vi "运维调试_五参数.vi"(11 "编号":string) -> ()   [LabVIEW 2016, in "斯坦道多参数.lvlib"]
uses:
  <vilib>/Utility/miscctls.llb/LVPointTypeDef.ctl
  <vilib>/Plasmionique/MB Master/MB_Master/MB_Master.lvclass
  <vilib>/Utility/config.llb/NI_LVConfig.lvlib
panel:
  in  "仪器参数":bool
  in  "参数设置选项卡":enum32{"选项卡 1", "选项卡 2"}(tab)
  in  "pH":bool
  in  "DO":bool
  in  "Turb":bool
  in  "Cond":bool
  in  "Temp":bool
  in  "叶绿素a启用":bool
  in  "藻密度":bool
  in  "pH探头选择":u16(ring) items=["YL型", "MQ型", "NAQ型"]
  in  "DO探头选择":u16(ring) items=["YL型", "MQ型", "NAQ型"]
  in  "电导率探头选择":u16(ring) items=["YL型", "MQ型", "NAQ型"]
  in  "浊度探头选择":u16(ring) items=["YL型", "MQ型", "NAQ型"]
  in  "叶绿素a探头选择":u16(ring) items=["YL型", "MQ型", "NAQ型"]
  in  "藻密度探头选择":u16(ring) items=["YL型", "MQ型", "NAQ型"]
  in  "ORP启用":bool
  in  "ORP探头选择":u16(ring) items=["YL型", "MQ型", "NAQ型"]
  in  "校准选择":T1
  out "模块版本号":string
  out "权限等级":string
  in  "水样测量时间":dbl caption="水样测量时间:"
  in  "打开modbus":bool
  out "选项卡控件":enum32{"选项卡 1", "选项卡 2"}(tab)
  in  "VISA资源名称":refnum<visa-resource-name> caption="串口"
  in  "IP":string="localhost" caption="IP:"
  in  "Port":u16=502 caption="Port:"
  in  "自动断线重连":bool=TRUE
  in  "连接方式":u16(ring) items=["Modbus RTU", "Modbus TCP"]
  in  "密码锁":bool
  in  "设置页返回":bool
  in  "周期设置":bool
  out "当前串口":string
  out "运行状态":enum16{"空闲", "水样测试", "标样核查"}(ring)
  in  "停止":bool
  in  "标样核查":bool
  in  "水样测试":bool
  in  "设置":bool
  in  "探头校正返回":bool
  in  "探头校正":bool
  out "检测值":T2
  # "请设置仪器连接方式"
  # "请选择要启用的参数"
  # "min"
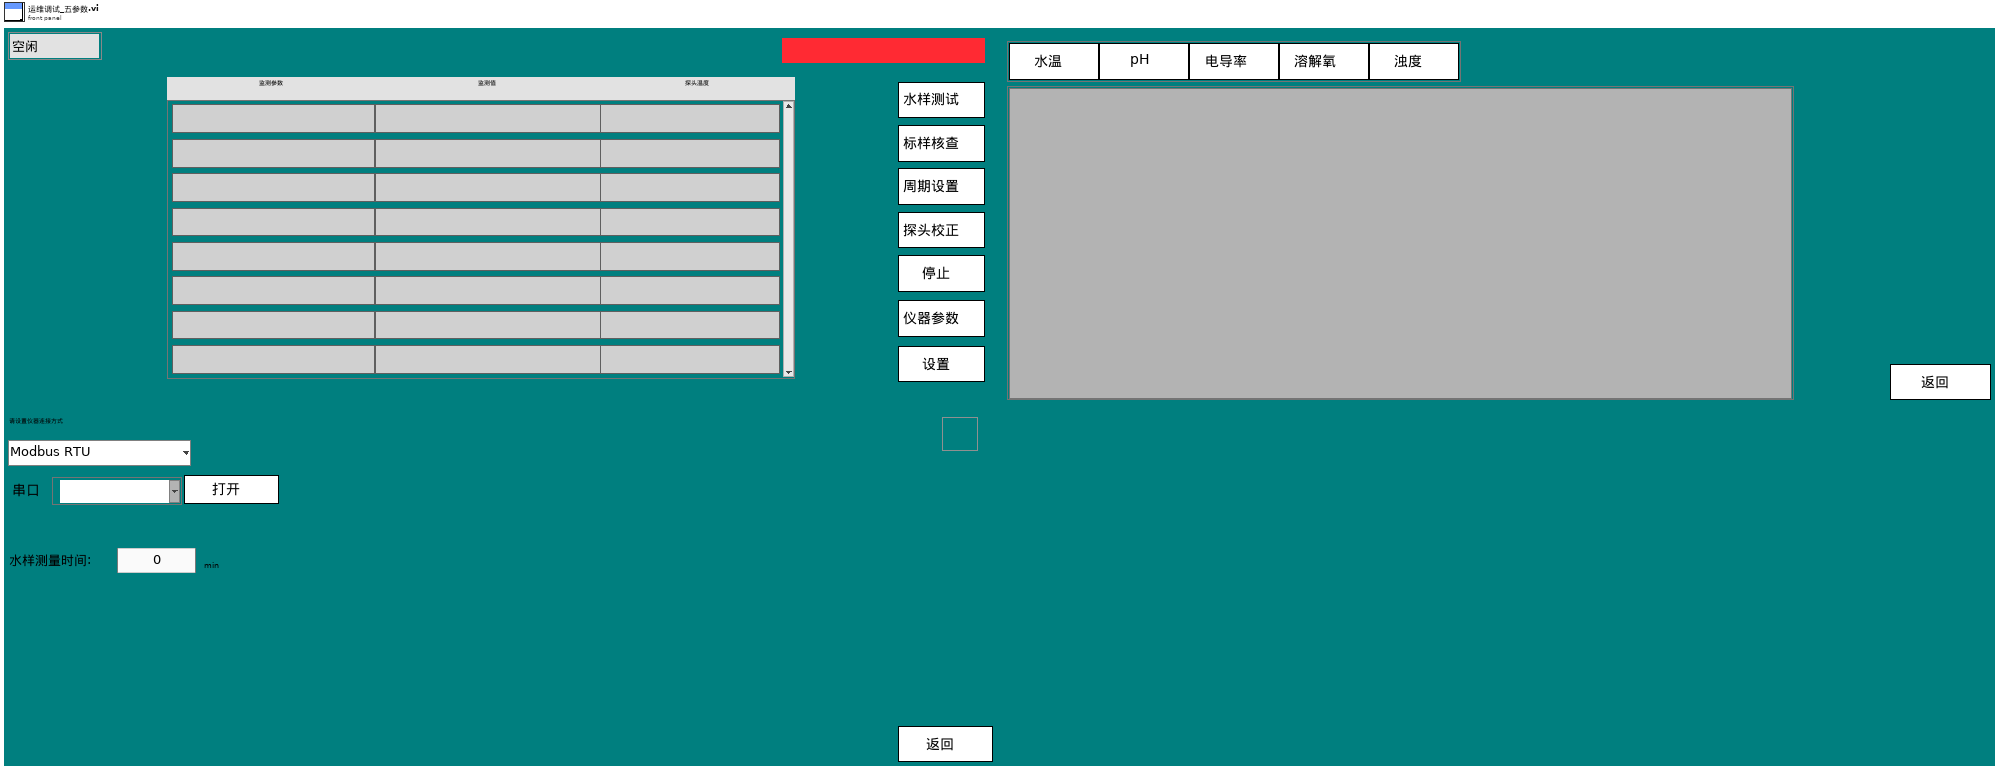
[diagram p1: front panel]
types:
  T1 = cluster{"水温校准":bool, "pH校准":bool, "电导率校准":bool, "溶解氧校准":bool, "浊度校准":bool, "叶绿素a校准":bool, "藻密度校准":bool, "ORP校准":bool}
  T2 = typedef "斯坦道多参数.lvlib/检测值.ctl" = cluster{"监测参数1":string, "浓度1":string, "探头温度1":string}[]
  T3 = typedef "LVPointTypeDef.ctl" = cluster{"Horizontal":i16, "Vertical":i16}
  T4 = cluster{"CH":u16, "监测值":dbl, "温度偏移修正值":sgl, "信号值":sgl}
  T5 = cluster{"温度测量值":sgl, "测量值":sgl, "温度偏移修正值":sgl, "信号值":sgl}
  T6 = cluster{"温度测量值":sgl, "DO%":sgl, "DOmg/L":sgl, "温度偏移修正值":sgl}
  T7 = cluster{"电极状态标志":u16, "电极型号标志":u16, "浊度测量值":sgl, "温度测量值":sgl, "浊度信号值":sgl, "浊度偏移修正值":sgl, "温度偏移修正值":sgl, "手动温度补偿值":sgl, "浊度电极零点":sgl, "浊度电极斜率":sgl, "第1点标准值记录":sgl, "第1点信号值记录":sgl, "第1点温度值记录":sgl, "第2点标准值记录":sgl, "第2点信号值记录":sgl, "第2点温度值记录":sgl, "命令滤波设定":u16, "温度模式":enum16{"ATC", "MTC"}, "生产批次":u16, "电极序号":u16, "串口地址":u16, "串口波特率":enum16{"9600", "19200", "115200"}, "串口校验位":enum16{"NONE", "ODD", "EVEN"}, "串口停止位":enum16{"1bit", "2bit"}, "第一点标准值":sgl, "第二点标准值":sgl, "第三点标准值":sgl}
  T8 = cluster{"电极状态标志":u16, "电极型号标志":u16, "溶解氧测量值":sgl, "温度测量值":sgl, "溶解氧饱和度值":sgl, "盐度补偿值":sgl, "大气压补偿值":sgl, "溶解氧偏移修正值":sgl, "温度偏移修正值":sgl, "手动温度补偿值":sgl, "溶解氧电极零点":sgl, "溶解氧电极斜率":sgl, "第1点标准值记录":sgl, "第1点信号值记录":sgl, "第1点温度值记录":sgl, "第2点标准值记录":sgl, "第2点信号值记录":sgl, "第2点温度值记录":sgl, "命令滤波设定":u16, "温度模式":enum16{"ATC", "MTC"}, "生产批次":u16, "电极序号":u16, "串口地址":u16, "串口波特率":enum16{"9600", "19200", "115200"}, "串口校验位":enum16{"NONE", "ODD", "EVEN"}, "串口停止位":enum16{"1bit", "2bit"}, "第一点标准值":sgl, "第二点标准值":sgl}
  T9 = cluster{"电极状态标志":u16, "电极型号标志":u16, "酸碱度测量值":sgl, "温度测量值":sgl, "酸碱度信号值":sgl, "温度信号值":sgl, "酸碱度偏移修正值":sgl, "温度偏移修正值":sgl, "手动温度补偿值":sgl, "酸碱度电极零点":sgl, "酸碱度电极斜率":sgl, "第1点标准值记录":sgl, "第1点信号值记录":sgl, "第1点温度值记录":sgl, "第2点标准值记录":sgl, "第2点信号值记录":sgl, "第2点温度值记录":sgl, "命令滤波设定":u16, "温度模式":enum16{"ATC", "MTC"}, "生产批次":u16, "电极序号":u16, "串口地址":u16, "串口波特率":enum16{"9600", "19200", "115200"}, "串口校验位":enum16{"NONE", "ODD", "EVEN"}, "串口停止位":enum16{"1bit", "2bit"}, "第一点标准值":sgl, "第二点标准值":sgl}
  T10 = cluster{"测量量程":dbl, "测量精度":dbl, "测量间隔":dbl, "消解温度":dbl, "消解时长":dbl, "空白校准时间":timestamp, "曲线截距":dbl, "曲线斜率":dbl, "测量检出限":dbl, "测量信号值":dbl, "线性相关系数":dbl, "二次多项式系数":dbl, "标样校准时间":timestamp, "稀释倍数":dbl, "三项式系数":dbl, "空白标定系数":dbl, "量程系数":dbl, "F0/ORPA":dbl, "F1/ORPB":dbl, "F2/ORPK":dbl, "F3":dbl, "F4":dbl, "F5":dbl, "F6":dbl, "F7":dbl, "X0/滴定数":dbl, "量程":dbl}
  T11 = cluster{"电极状态标志":u16, "电极型号标志":u16, "电导率测量值":sgl, "温度测量值":sgl, "电导率信号值":sgl, "温度信号值":sgl, "温度补偿系数":sgl, "电导率偏移修正值":sgl, "温度偏移修正值":sgl, "手动温度补偿值":sgl, "电导率电极零点":sgl, "电导率电极斜率":sgl, "命令滤波设定":u16, "温度模式":enum16{"ATC", "MTC"}, "生产批次":u16, "电极序号":u16, "串口地址":u16, "串口波特率":enum16{"9600", "19200", "115200"}, "串口校验位":enum16{"NONE", "ODD", "EVEN"}, "串口停止位":enum16{"1bit", "2bit"}, "第一点标准值":sgl, "第二点标准值":sgl}
  T12 = enum8{"Enabled", "Disabled", "Disabled and Grayed Out"}
  T13 = cluster{"pH探头选择":u16, "DO探头选择":u16, "电导率探头选择":u16, "浊度探头选择":u16, "叶绿素a探头选择":u16, "蓝绿藻探头选择":u16, "orp探头选择":u16}
  T14 = cluster{"监测参数1":string, "浓度1":string, "探头温度1":string}[]
  T15 = cluster{"周期设置类型":enum16{"定点启动", "间隔启动"}, "定时功能启用":bool, "定时间隔":u32, "24H周期设置":bool[]}
  T16 = enum32{"Bad", "Idle", "Run top level", "Running"}
  T17 = typedef "LVDateTimeRec.ctl" = cluster{"秒数的小数部分":dbl, "秒":i32, "分":i32, "时":i32, "日":i32, "月":i32, "年":i32, "天数（周）":i32, "天数（年）":i32, "DST":i32}
  T18 = cluster{"Major":u16, "Minor":u16, "Fix":u16, "Build":u16}
  T19 = typedef "NI_LVConfig.lvlib/Config Data RefNum.ctl" = refnum<k1>
  T20 = cluster{"baud rate (bps)":u32, "stop bits":u16, "parity":u16, "flow control":u16, "timeout":u32, "retries":i32}
  T21 = cluster{"pH校准VI引用句柄":refnum<vi>, "DO校准VI引用句柄":refnum<vi>, "COND校准VI引用句柄":refnum<vi>, "TURB校准VI引用句柄":refnum<vi>, "CHLA校准VI引用句柄":refnum<vi>, "BGA校准VI引用句柄":refnum<vi>, "ORP校准VI引用句柄":refnum<vi>}
  T22 = cluster{"测量量程":dbl, "测量精度":dbl, "测量间隔":dbl, "消解温度":dbl, "消解时长":dbl, "空白校准时间":timestamp, "曲线截距":dbl, "曲线斜率":dbl, "测量检出限":dbl, "测量信号值":dbl, "线性相关系数":dbl, "二次多项式系数":dbl, "标样校准时间":timestamp, "稀释倍数":dbl, "三项式系数":dbl, "空白标定系数":dbl, "量程系数":dbl, "F0/ORPA":dbl, "F1/ORPB":dbl, "F2/ORPK":dbl, "F3":dbl, "F4":dbl, "F5":dbl, "F6":dbl, "F7":dbl, "X0/滴定数":dbl, "量程":dbl}[]
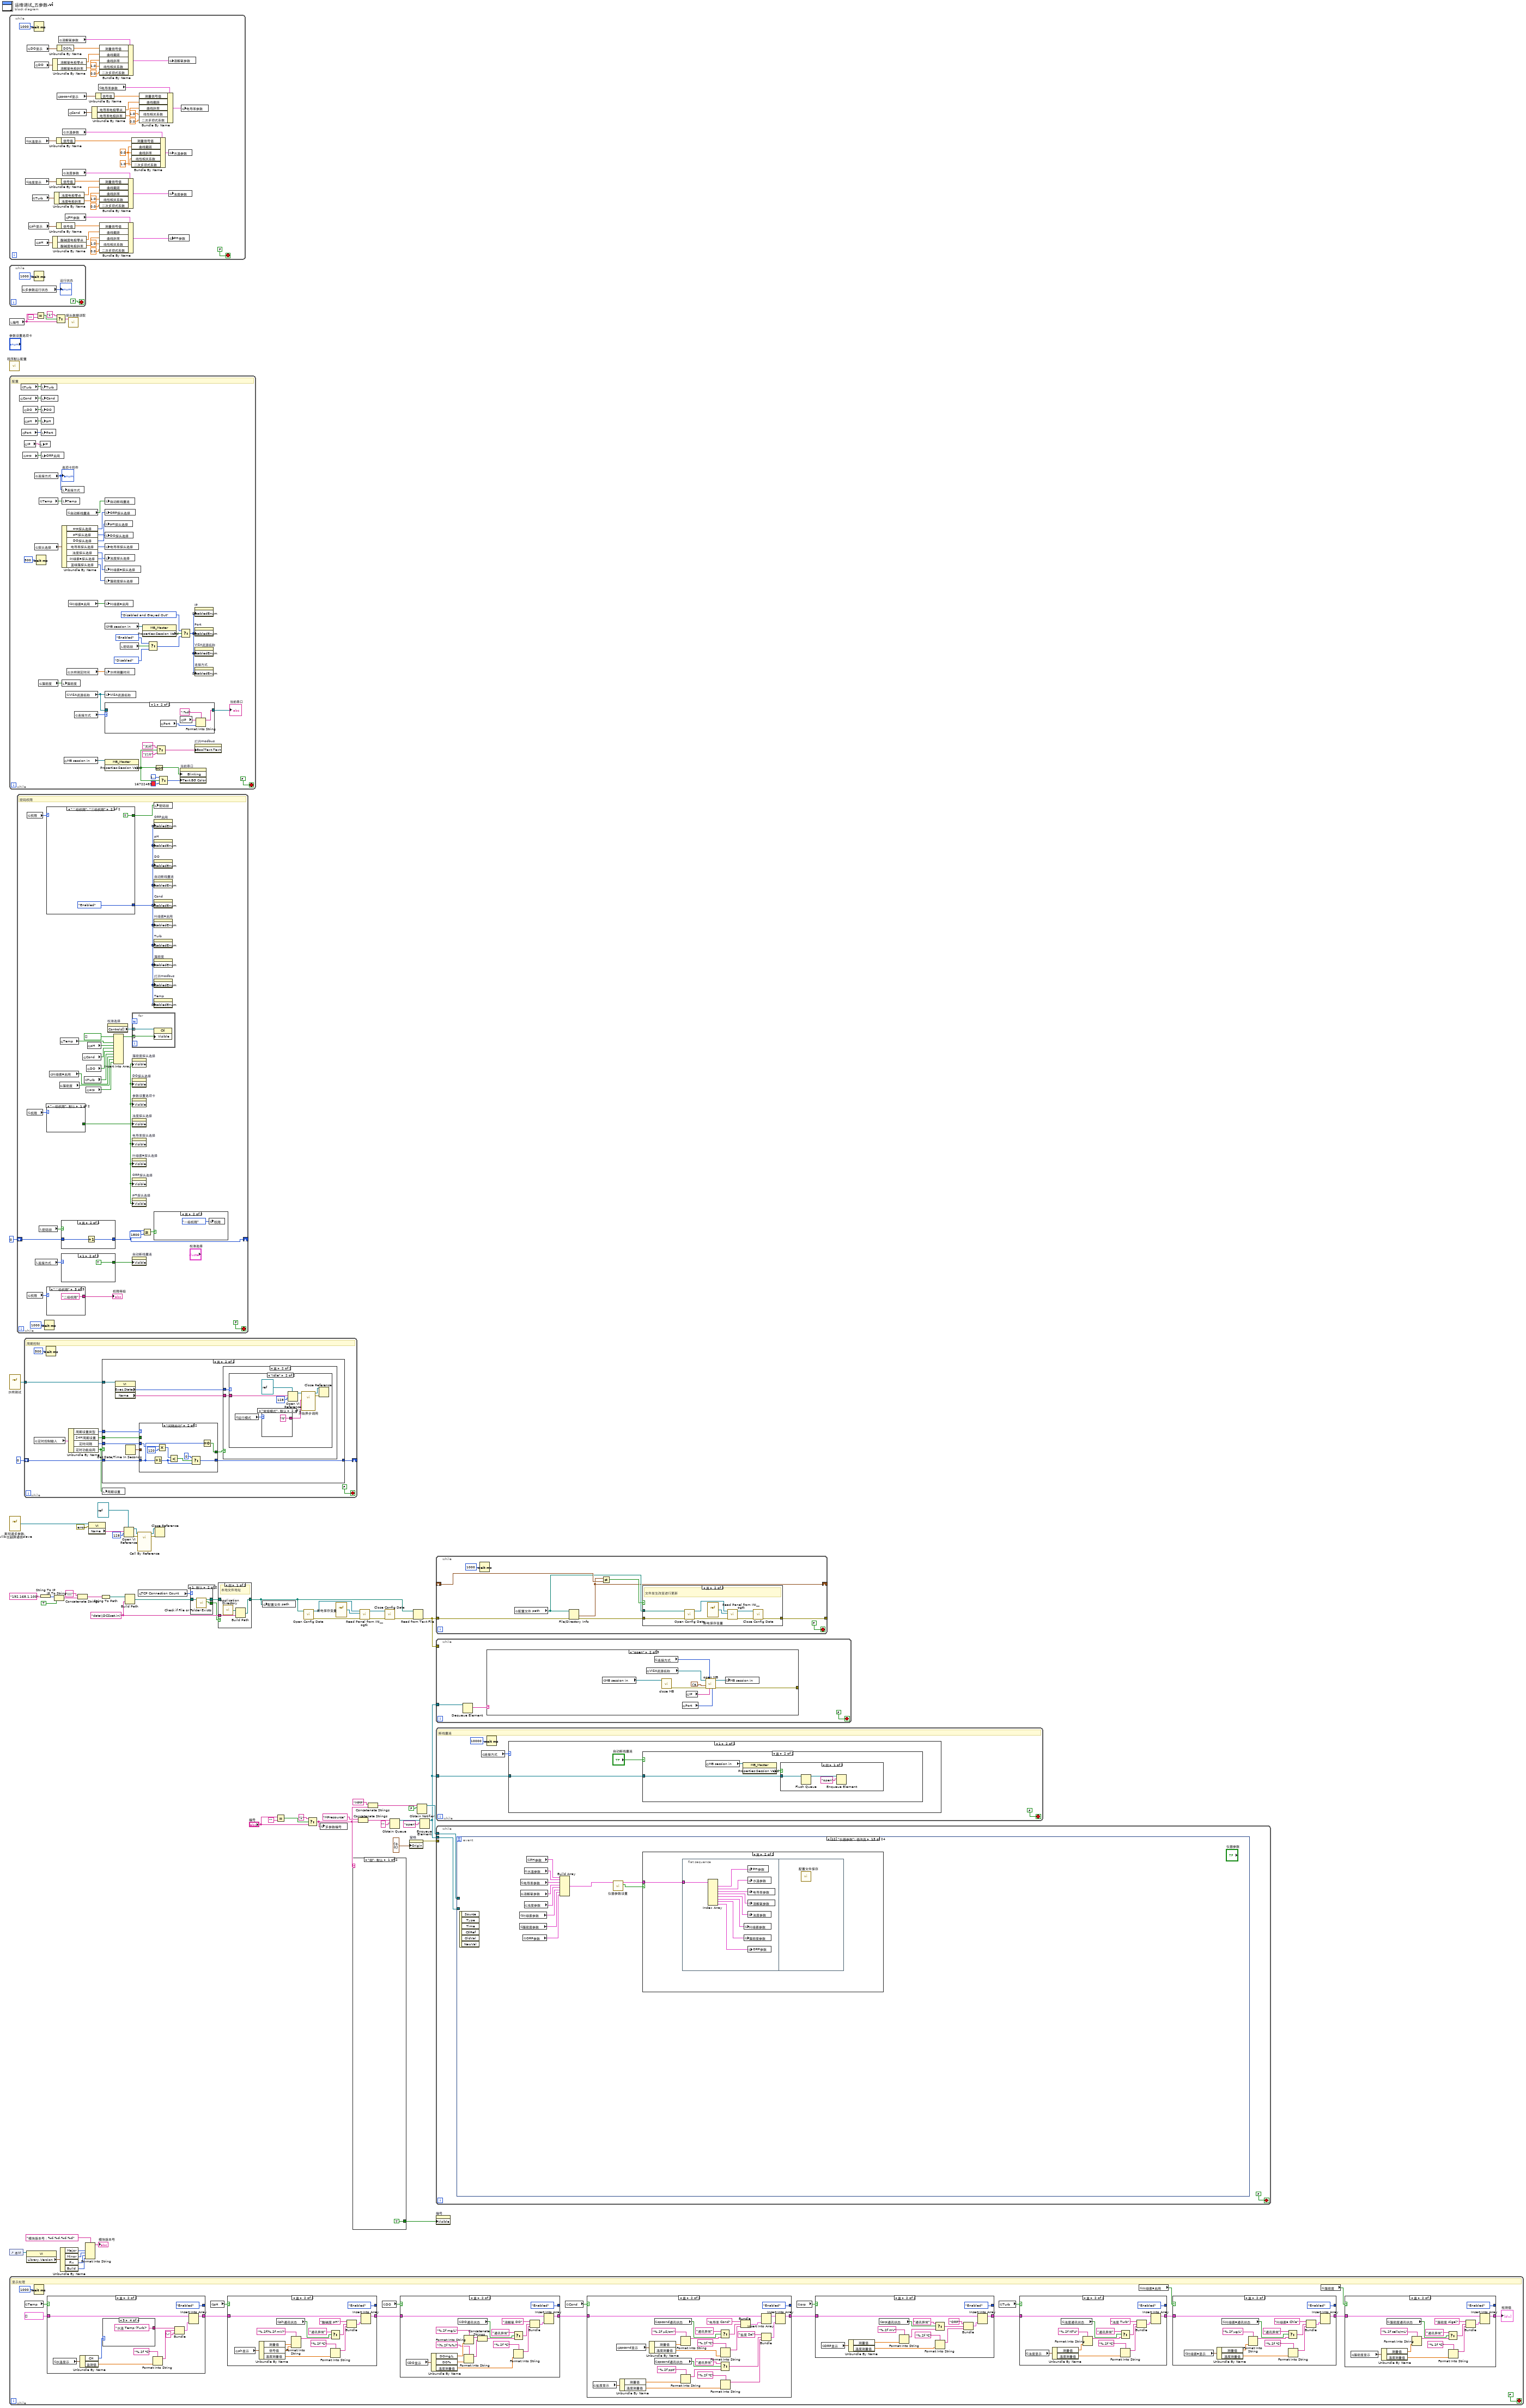
[diagram p0: block diagram]
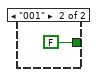
[diagram p3: hidden frame]
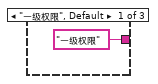
[diagram p12: hidden frame]
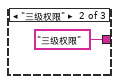
[diagram p13: hidden frame]
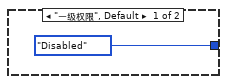
[diagram p14: hidden frame]
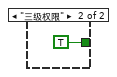
[diagram p15: hidden frame]
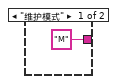
[diagram p19: hidden frame]
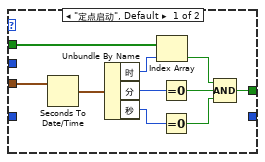
[diagram p20: hidden frame]
diagram:
  w34 = "data\\DCSset.ini" ("名称或相对路径")
  n1 = while {
    stop <- FALSE stop-if-true
    w64 = 0.0 ("二次多项式系数")
    n2 = global read "多参数全局变量.vi" "水温显示"() -> (w85:T4)
    n3 = global read "多参数全局变量.vi" "浊度显示"() -> (w67:T5)
    n4 = global read "多参数全局变量.vi" "DO显示"() -> (w99:T6)
    n5 = global read "多参数全局变量.vi" "ph显示"() -> (w94:T5)
    n6 = global read "国弘过程全局变量.vi" "Turb"() -> (w69:T7)
    n7 = Wait (ms)(milliseconds to wait=u32 1000 ("等待时间（毫秒）")) -> ()  [unwired: 1 out]
    n8 = global read "国弘过程全局变量.vi" "DO"() -> (w101:T8)
    n9 = global read "国弘过程全局变量.vi" "pH"() -> (w92:T9)
    n10 = Unbundle By Name(w101) -> ("溶解氧电极零点"=w102:sgl, "溶解氧电极斜率"=w103:sgl)
    n11 = Unbundle By Name(w92) -> ("酸碱度电极零点"=w91:sgl, "酸碱度电极斜率"=w90:sgl)
    n12 = Unbundle By Name(w69) -> ("浊度电极零点"=w70:sgl, "浊度电极斜率"=w71:sgl)
    n13 = Unbundle By Name(w85) -> ("信号值"=w86:sgl)
    n14 = Unbundle By Name(w67) -> ("信号值"=w68:sgl)
    n15 = Unbundle By Name(w94) -> ("信号值"=w93:sgl)
    n16 = Unbundle By Name(w99) -> ("DO%"=w100:sgl)
    n17 = global read "多参数全局变量.vi" "spcond显示"() -> (w80:T5)
    n18 = global read "断电保存变量.vi" "溶解氧参数"() -> (w97:T10)
    n19 = global read "断电保存变量.vi" "水温参数"() -> (w83:T10)
    n20 = global read "断电保存变量.vi" "浊度参数"() -> (w65:T10)
    n21 = global read "断电保存变量.vi" "PH参数"() -> (w96:T10)
    n22 = global read "国弘过程全局变量.vi" "Cond"() -> (w78:T11)
    n23 = Unbundle By Name(w78) -> ("电导率电极零点"=w77:sgl, "电导率电极斜率"=w76:sgl)
    n24 = Unbundle By Name(w80) -> ("信号值"=w79:sgl)
    n25 = global read "断电保存变量.vi" "电导率参数"() -> (w82:T10)
    n26 = Bundle By Name(cluster=w97, "测量信号值"=w100, "曲线截距"=w102, "曲线斜率"=w103, "线性相关系数"=1.0, "二次多项式系数"=0.0) -> (w98:T10)
    n27 = Bundle By Name(cluster=w65, "测量信号值"=w68, "曲线截距"=w70, "曲线斜率"=w71, "线性相关系数"=1.0, "二次多项式系数"=0.0) -> (w66:T10)
    n28 = Bundle By Name(cluster=w96, "测量信号值"=w93, "曲线截距"=w91, "曲线斜率"=w90, "线性相关系数"=1.0, "二次多项式系数"=0.0) -> (w95:T10)
    n29 = Bundle By Name(cluster=w83, "测量信号值"=w86, "曲线截距"=w64, "曲线斜率"=w64, "线性相关系数"=1.0, "二次多项式系数"=w64) -> (w84:T10)
    n30 = Bundle By Name(cluster=w82, "测量信号值"=w79, "曲线截距"=w77, "曲线斜率"=w76, "线性相关系数"=1.0, "二次多项式系数"=0.0) -> (w81:T10)
    n31 = global write "断电保存变量.vi" "溶解氧参数"(w98) -> ()
    n32 = global write "断电保存变量.vi" "水温参数"(w84) -> ()
    n33 = global write "断电保存变量.vi" "浊度参数"(w66) -> ()
    n34 = global write "断电保存变量.vi" "PH参数"(w95) -> ()
    n35 = global write "断电保存变量.vi" "电导率参数"(w81) -> ()
  }
  n36 = while {
    stop <- FALSE stop-if-true
    n37 = global read "多参数全局变量.vi" "多参数运行状态"() -> (→"运行状态":u16)
    n38 = Wait (ms)(milliseconds to wait=u32 1000 ("等待时间（毫秒）")) -> ()  [unwired: 1 out]
  }
  n39 = local read "编号"() -> (w10:string)
  n40 = call "程序默认配置.vi"() -> ()  [unwired: 11 in, 1 out]
  n41 = while {
    stop <- FALSE stop-if-true
    # "配置"
    n42 = global read "断电保存变量.vi" "Cond"() -> (w149:bool)
    n43 = global read "断电保存变量.vi" "Turb"() -> (w148:bool)
    n44 = global read "断电保存变量.vi" "Port"() -> (w127:u16)
    n45 = global read "断电保存变量.vi" "orp"() -> (w112:bool)
    n46 = global read "断电保存变量.vi" "DO"() -> (w150:bool)
    n47 = global read "断电保存变量.vi" "pH"() -> (w151:bool)
    n48 = global read "断电保存变量.vi" "IP"() -> (w128:string)
    n49 = global read "断电保存变量.vi" "连接方式"() -> (w120:u16)
    "选项卡控件" <- w120
    n50 = global read "断电保存变量.vi" "探头选择"() -> (w138:T13)
    n51 = Wait (ms)(milliseconds to wait=u32 500 ("等待时间（毫秒）")) -> ()  [unwired: 1 out]
    n52 = global read "断电保存变量.vi" "藻密度"() -> (w146:bool)
    n53 = global read "断电保存变量.vi" "Temp"() -> (w152:bool)
    n54 = local write "IP"(w128) -> ()
    n55 = local write "Turb"(w148) -> ()
    n56 = local write "Cond"(w149) -> ()
    n57 = local write "DO"(w150) -> ()
    n58 = local write "pH"(w151) -> ()
    n59 = local write "Port"(w127) -> ()
    n60 = local write "ORP启用"(w112) -> ()
    n61 = local write "连接方式"(w120) -> ()
    n62 = local write "Temp"(w152) -> ()
    n63 = Unbundle By Name(w138) -> ("orp探头选择"=w111:u16, "pH探头选择"=w121:u16, "DO探头选择"=w137:u16, "电导率探头选择"=w136:u16, "浊度探头选择"=w135:u16, "叶绿素a探头选择"=w134:u16, "蓝绿藻探头选择"=w133:u16)
    n64 = local write "藻密度"(w146) -> ()
    n65 = global read "多参数全局变量.vi" "MB session in"() -> (w142:refnum<class "MB_Master.lvclass">)
    n66 = global read "断电保存变量.vi" "VISA资源名称"() -> (w124:refnum<visa-resource-name>)
    n67 = global read "断电保存变量.vi" "自动断线重连"() -> (w115:bool)
    n68 = global read "断电保存变量.vi" "水样测定时间"() -> (w114:dbl)
    n69 = global read "断电保存变量.vi" "叶绿素a启用"() -> (w147:bool)
    n70 = global read "断电保存变量.vi" "连接方式"() -> (w125:u16)
    n71 = local write "自动断线重连"(w115) -> ()
    n72 = local write "ORP探头选择"(w111) -> ()
    n73 = local write "pH探头选择"(w121) -> ()
    n74 = local write "DO探头选择"(w137) -> ()
    n75 = local write "电导率探头选择"(w136) -> ()
    n76 = local write "浊度探头选择"(w135) -> ()
    n77 = local write "叶绿素a探头选择"(w134) -> ()
    n78 = local write "藻密度探头选择"(w133) -> ()
    n79 = local write "叶绿素a启用"(w147) -> ()
    n80 = global read "多参数全局变量.vi" "MB session in"() -> (w145:refnum<class "MB_Master.lvclass">)
    n81 = local write "水样测量时间"(w114) -> ()
    n82 = local write "VISA资源名称"(w124) -> ()
    n83 = case shown="1" w125 {
      tunnel: w124 -> [w154 _]
      tunnel: [w154 w155] -> w123
      frame 0, Default {
      }
      frame 1 {
        n84 = global read "断电保存变量.vi" "Port"() -> (w156:u16)
        n85 = global read "断电保存变量.vi" "IP"() -> (w158:string)
        n86 = Format Into String(format string=":%d" ("格式字符串"), initial string=w158, w156) -> (resulting string=w155:string)  [unwired: 1 in, 1 out]
      }
    }
    "当前串口" <- w123
    n87 = property class="MB_Master"(reference=w142) -> ("Properties:Session Valid"=w119:bool)  [unwired: 1 in, 2 out]
    n88 = local read "密码锁"() -> (w132:bool)
    n89 = property class="MB_Master"(reference=w145) -> ("Properties:Session Valid"=w144:bool)  [unwired: 1 in, 2 out]
    n90 = Select(t=T12."Enabled" ("f"), s=w132, f=T12."Disabled") -> (s? t:f=w130:T12)
    n91 = Not(x=w119) -> (.not. x?=w122:bool)
    n92 = Select(t="关闭" ("布尔文本.文本"), s=w119, f="打开" ("布尔文本.文本")) -> (s? t:f=w139:string)
    n93 = Select(t=u32 16777216, s=w119, f=u32 16722483) -> (s? t:f=w116:u32)
    n94 = property on="当前串口" class="Str"("Blinking"=w122, "Text.BG Color"=w116) -> ()  [unwired: 2 in, 2 out]
    n95 = Select(t=T12."Disabled and Grayed Out" ("禁用"), s=w144, f=w130) -> (s? t:f=w126:T12)
    n96 = property on="IP" class="Str"("DisabledEnum"=w126) -> ()  [unwired: 2 in, 2 out]
    n97 = property on="Port" class="DigNum (严格)"("DisabledEnum"=w126) -> ()  [unwired: 2 in, 2 out]
    n98 = property on="VISA资源名称" class="VISAName"("DisabledEnum"=w126) -> ()  [unwired: 2 in, 2 out]
    n99 = property on="连接方式" class="Ring (严格)"("DisabledEnum"=w126) -> ()  [unwired: 2 in, 2 out]
    n100 = property on="打开modbus" class="Bool"("BoolText.Text"=w139) -> ()  [unwired: 2 in, 2 out]
  }
  n101 = vi-ref "水样测试.vi"() -> (w53:refnum<vi>)
  n102 = vi-ref "斯坦道多参数.lvlib:主副屏通信slave.vi"() -> (w35:refnum<vi>)
  n103 = control-ref of="本VI"() -> (w26:refnum<vi>)
  n104 = while {
    stop <- FALSE stop-if-true
    # "显示处理"
    n105 = global read "断电保存变量.vi" "Temp"() -> (w175:bool)
    n106 = Wait (ms)(milliseconds to wait=u32 1000 ("等待时间（毫秒）")) -> ()  [unwired: 1 out]
    n107 = case shown="真" w175 {
      tunnel: [w316 w321] -> w172
      tunnel: T14 [] ("数组") -> [w316 w322]
      tunnel: [T12."Disabled and Grayed Out" ("禁用") T12."Enabled" ("禁用")] -> _
      frame False {
      }
      frame True {
        n108 = global read "多参数全局变量.vi" "水温显示"() -> (w319:T4)
        n109 = Unbundle By Name(w319) -> ("CH"=w318:u16, "监测值"=w317:dbl)
        n110 = case shown="3" w318 {
          tunnel: ["水温 Temp (pH)" ("监测参数1") "水温 Temp (Cond)" ("监测参数1") "水温 Temp (DO)" ("监测参数1") "水温 Temp (Turb)" ("监测参数1")] -> w326
          frame 0, Default {
          }
          frame 1 {
          }
          frame 2 {
          }
          frame 3 {
          }
        }
        n111 = Format Into String(format string="%.2f ℃" ("格式字符串"), w317) -> (resulting string=w325:string)  [unwired: 2 in, 1 out]
        n112 = Bundle("监测参数1"=w326, w325, "探头温度1"="-") -> (w323:cluster{"监测参数1":string, string, "探头温度1":string})  [unwired: 1 in]
        n113 = Insert Into Array(array=w322, new element=w323) -> (w321:T14)  [unwired: 1 in]
      }
    }
    n114 = global read "断电保存变量.vi" "pH"() -> (w173:bool)
    n115 = case shown="真" w173 {
      tunnel: [w298 w306] -> w170
      tunnel: w172 -> [w298 w308]
      tunnel: [T12."Disabled and Grayed Out" ("禁用") T12."Enabled" ("禁用")] -> _
      frame False {
      }
      frame True {
        n116 = global read "多参数全局变量.vi" "ph显示"() -> (w304:T5)
        n117 = Unbundle By Name(w304) -> ("测量值"=w314:sgl, "信号值"=w299:sgl, "温度测量值"=w312:sgl)
        n118 = global read "多参数全局变量.vi" "ph通讯状态"() -> (w302:bool)
        n119 = Format Into String(format string="%.2f(%.2f mV)" ("格式字符串"), w314, w299) -> (resulting string=w301:string)  [unwired: 2 in, 1 out]
        n120 = Select(t="通讯异常" ("格式字符串"), s=w302, f=w301) -> (s? t:f=w300:string)
        n121 = Format Into String(format string="%.2f ℃" ("格式字符串"), w312) -> (resulting string=w310:string)  [unwired: 2 in, 1 out]
        n122 = Bundle("监测参数2"="酸碱度 pH", "格式字符串"=w300, w310) -> (w307:cluster{"监测参数2":string, "格式字符串":string, string})  [unwired: 1 in]
        n123 = Insert Into Array(array=w308, new element=w307) -> (w306:T14)  [unwired: 1 in]
      }
    }
    n124 = global read "断电保存变量.vi" "DO"() -> (w171:bool)
    n125 = case shown="真" w171 {
      tunnel: [w277 w284] -> w167
      tunnel: w170 -> [w277 w285]
      tunnel: [T12."Disabled and Grayed Out" ("禁用") T12."Enabled" ("禁用")] -> _
      frame False {
      }
      frame True {
        n126 = global read "多参数全局变量.vi" "DO显示"() -> (w282:T6)
        n127 = Unbundle By Name(w282) -> ("DOmg/L"=w293:sgl, "DO%"=w291:sgl, "温度测量值"=w295:sgl)
        n128 = global read "多参数全局变量.vi" "DO通讯状态"() -> (w280:bool)
        n129 = Format Into String(format string="%.2f mg/L" ("格式字符串"), w293) -> (resulting string=w290:string)  [unwired: 2 in, 1 out]
        n130 = Format Into String(format string="(%.2f %%)" ("格式字符串"), w291) -> (resulting string=w289:string)  [unwired: 2 in, 1 out]
        n131 = Concatenate Strings(w290, w289) -> (w279:string)
        n132 = Select(t="通讯异常" ("格式字符串"), s=w280, f=w279) -> (s? t:f=w278:string)
        n133 = Format Into String(format string="%.2f ℃" ("格式字符串"), w295) -> (resulting string=w287:string)  [unwired: 2 in, 1 out]
        n134 = Bundle("监测参数2"="溶解氧 DO", "格式字符串"=w278, w287) -> (w286:cluster{"监测参数2":string, "格式字符串":string, string})  [unwired: 1 in]
        n135 = Insert Into Array(array=w285, new element=w286) -> (w284:T14)  [unwired: 1 in]
      }
    }
    n136 = global read "断电保存变量.vi" "Cond"() -> (w169:bool)
    n137 = case shown="真" w169 {
      tunnel: w167 -> [w247 w271]
      tunnel: [w247 w260] -> w159
      tunnel: [T12."Disabled and Grayed Out" ("禁用") T12."Enabled" ("禁用")] -> _
      frame False {
      }
      frame True {
        n138 = global read "多参数全局变量.vi" "盐度显示"() -> (w253:T5)
        n139 = global read "多参数全局变量.vi" "spcond显示"() -> (w268:T5)
        n140 = Unbundle By Name(w253) -> ("测量值"=w254:sgl, "温度测量值"=w255:sgl)
        n141 = Unbundle By Name(w268) -> ("测量值"=w267:sgl, "温度测量值"=w266:sgl)
        n142 = global read "多参数全局变量.vi" "spcond通讯状态"() -> (w264:bool)
        n143 = global read "多参数全局变量.vi" "spcond通讯状态"() -> (w257:bool)
        n144 = Format Into String(format string="%.2f μS/cm" ("格式字符串"), w267) -> (resulting string=w263:string)  [unwired: 2 in, 1 out]
        n145 = Format Into String(format string="%.2f ppt" ("格式字符串"), w254) -> (resulting string=w258:string)  [unwired: 2 in, 1 out]
        n146 = Select(t="通讯异常" ("格式字符串"), s=w264, f=w263) -> (s? t:f=w262:string)
        n147 = Select(t="通讯异常" ("格式字符串"), s=w257, f=w258) -> (s? t:f=w259:string)
        n148 = Format Into String(format string="%.2f ℃" ("格式字符串"), w266) -> (resulting string=w272:string)  [unwired: 2 in, 1 out]
        n149 = Format Into String(format string="%.2f ℃" ("格式字符串"), w255) -> (resulting string=w252:string)  [unwired: 2 in, 1 out]
        n150 = Bundle("监测参数2"="电导率 Cond", "格式字符串"=w262, w272) -> (w270:cluster{"监测参数2":string, "格式字符串":string, string})  [unwired: 1 in]
        n151 = Insert Into Array(array=w271, new element=w270) -> (w261:T14)  [unwired: 1 in]
        n152 = Bundle("监测参数2"="盐度 Sal", "格式字符串"=w259, w252) -> (w248:cluster{"监测参数2":string, "格式字符串":string, string})  [unwired: 1 in]
        n153 = Insert Into Array(array=w261, new element=w248) -> (w260:T14)  [unwired: 1 in]
      }
    }
    n154 = global read "断电保存变量.vi" "orp"() -> (w161:bool)
    n155 = case shown="真" w161 {
      tunnel: w159 -> [w179 w190]
      tunnel: [w179 w188] -> w160
      tunnel: [T12."Disabled and Grayed Out" ("禁用") T12."Enabled" ("禁用")] -> _
      frame False {
      }
      frame True {
        n156 = global read "多参数全局变量.vi" "ORP显示"() -> (w186:T5)
        n157 = Unbundle By Name(w186) -> ("测量值"=w185:sgl, "温度测量值"=w184:sgl)
        n158 = global read "多参数全局变量.vi" "orp通讯状态"() -> (w182:bool)
        n159 = Format Into String(format string="%.2f mV" ("格式字符串"), w185) -> (resulting string=w181:string)  [unwired: 2 in, 1 out]
        n160 = Select(t="通讯异常" ("格式字符串"), s=w182, f=w181) -> (s? t:f=w180:string)
        n161 = Format Into String(format string="%.2f ℃" ("格式字符串"), w184) -> (resulting string=w191:string)  [unwired: 2 in, 1 out]
        n162 = Bundle("监测参数2"="ORP", "格式字符串"=w180, w191) -> (w189:cluster{"监测参数2":string, "格式字符串":string, string})  [unwired: 1 in]
        n163 = Insert Into Array(array=w190, new element=w189) -> (w188:T14)  [unwired: 1 in]
      }
    }
    n164 = global read "断电保存变量.vi" "Turb"() -> (w168:bool)
    n165 = case shown="真" w168 {
      tunnel: w160 -> [w230 w241]
      tunnel: [w230 w239] -> w166
      tunnel: [T12."Disabled and Grayed Out" ("禁用") T12."Enabled" ("禁用")] -> _
      frame False {
      }
      frame True {
        n166 = global read "多参数全局变量.vi" "浊度显示"() -> (w237:T5)
        n167 = Unbundle By Name(w237) -> ("测量值"=w236:sgl, "温度测量值"=w235:sgl)
        n168 = global read "多参数全局变量.vi" "浊度通讯状态"() -> (w233:bool)
        n169 = Format Into String(format string="%.2f NTU" ("格式字符串"), w236) -> (resulting string=w232:string)  [unwired: 2 in, 1 out]
        n170 = Select(t="通讯异常" ("格式字符串"), s=w233, f=w232) -> (s? t:f=w231:string)
        n171 = Format Into String(format string="%.2f ℃" ("格式字符串"), w235) -> (resulting string=w243:string)  [unwired: 2 in, 1 out]
        n172 = Bundle("监测参数2"="浊度 Turb", "格式字符串"=w231, w243) -> (w240:cluster{"监测参数2":string, "格式字符串":string, string})  [unwired: 1 in]
        n173 = Insert Into Array(array=w241, new element=w240) -> (w239:T14)  [unwired: 1 in]
      }
    }
    n174 = global read "断电保存变量.vi" "叶绿素a启用"() -> (w165:bool)
    n175 = case shown="真" w165 {
      tunnel: w166 -> [w213 w224]
      tunnel: [w213 w222] -> w163
      tunnel: [T12."Disabled and Grayed Out" ("禁用") T12."Enabled" ("禁用")] -> _
      frame False {
      }
      frame True {
        n176 = global read "多参数全局变量.vi" "叶绿素a显示"() -> (w218:T5)
        n177 = Unbundle By Name(w218) -> ("测量值"=w221:sgl, "温度测量值"=w220:sgl)
        n178 = global read "多参数全局变量.vi" "叶绿素a通讯状态"() -> (w216:bool)
        n179 = Format Into String(format string="%.2f μg/L" ("格式字符串"), w221) -> (resulting string=w215:string)  [unwired: 2 in, 1 out]
        n180 = Select(t="通讯异常" ("格式字符串"), s=w216, f=w215) -> (s? t:f=w214:string)
        n181 = Format Into String(format string="%.2f ℃" ("格式字符串"), w220) -> (resulting string=w226:string)  [unwired: 2 in, 1 out]
        n182 = Bundle("监测参数2"="叶绿素a Chla", "格式字符串"=w214, w226) -> (w223:cluster{"监测参数2":string, "格式字符串":string, string})  [unwired: 1 in]
        n183 = Insert Into Array(array=w224, new element=w223) -> (w222:T14)  [unwired: 1 in]
      }
    }
    n184 = global read "断电保存变量.vi" "藻密度"() -> (w164:bool)
    n185 = case shown="真" w164 {
      tunnel: w163 -> [w196 w207]
      tunnel: [w196 w205] -> w162
      tunnel: [T12."Disabled and Grayed Out" ("禁用") T12."Enabled" ("禁用")] -> _
      frame False {
      }
      frame True {
        n186 = global read "多参数全局变量.vi" "藻密度显示"() -> (w201:T5)
        n187 = Unbundle By Name(w201) -> ("测量值"=w204:sgl, "温度测量值"=w203:sgl)
        n188 = global read "多参数全局变量.vi" "藻密度通讯状态"() -> (w199:bool)
        n189 = Format Into String(format string="%.2f cells/mL" ("格式字符串"), w204) -> (resulting string=w198:string)  [unwired: 2 in, 1 out]
        n190 = Select(t="通讯异常" ("格式字符串"), s=w199, f=w198) -> (s? t:f=w197:string)
        n191 = Format Into String(format string="%.2f ℃" ("格式字符串"), w203) -> (resulting string=w209:string)  [unwired: 2 in, 1 out]
        n192 = Bundle("监测参数2"="藻密度 Algal", "格式字符串"=w197, w209) -> (w206:cluster{"监测参数2":string, "格式字符串":string, string})  [unwired: 1 in]
        n193 = Insert Into Array(array=w207, new element=w206) -> (w205:T14)  [unwired: 1 in]
      }
    }
    "检测值" <- w162
  }
  n194 = while {
    shift-right: [w354] -> _
    shift-left: u32 0 ("等待时间（毫秒）") -> [w355]
    stop <- FALSE stop-if-true
    # "密码权限"
    n195 = global read "多参数全局变量.vi" "权限"() -> (w345:enum16{"一级权限", "二级权限", "三级权限"})
    n196 = global read "多参数全局变量.vi" "权限"() -> (w346:enum16{"一级权限", "二级权限", "三级权限"})
    n197 = global read "多参数全局变量.vi" "权限"() -> (w347:enum16{"一级权限", "二级权限", "三级权限"})
    n198 = local read "连接方式"() -> (w351:u16)
    n199 = local read "密码锁"() -> (w356:bool)
    n200 = Wait (ms)(milliseconds to wait=u32 1000 ("等待时间（毫秒）")) -> ()  [unwired: 1 out]
    n201 = case shown="\"二级权限\", \"三级权限\"" w345 {
      tunnel: [T12."Disabled" ("禁用") T12."Enabled" ("禁用")] -> w349
      tunnel: [_ TRUE ("可见")] -> w344
      frame "一级权限", Default {
      }
      frame "二级权限", "三级权限" {
      }
    }
    n202 = case shown="\"一级权限\", 默认" w346 {
      tunnel: [_ TRUE ("可见")] -> w332
      frame "一级权限", Default {
      }
      frame "三级权限" {
      }
    }
    n203 = case shown="\"二级权限\"" w347 {
      tunnel: ["一级权限" ("权限等级") "三级权限" ("权限等级") "二级权限" ("权限等级")] -> w348
      frame "一级权限", Default {
      }
      frame "三级权限" {
      }
      frame "二级权限" {
      }
    }
    "权限等级" <- w348
    n204 = global read "断电保存变量.vi" "叶绿素a启用"() -> (w336:bool)
    n205 = global read "断电保存变量.vi" "藻密度"() -> (w335:bool)
    n206 = global read "断电保存变量.vi" "Temp"() -> (w342:bool)
    n207 = case shown="真" w356 {
      tunnel: w355 -> [_ w364]
      tunnel: [_ w363] -> w354
      frame False {
      }
      frame True {
        n208 = Increment(x=w364) -> (x+1=w363:u32)
      }
    }
    n209 = case shown="1" w351 {
      tunnel: [_ TRUE ("可见")] -> w350
      frame 0, Default {
      }
      frame 1 {
      }
    }
    n210 = global read "断电保存变量.vi" "Cond"() -> (w339:bool)
    n211 = global read "断电保存变量.vi" "Turb"() -> (w337:bool)
    n212 = global read "断电保存变量.vi" "orp"() -> (w334:bool)
    n213 = global read "断电保存变量.vi" "DO"() -> (w338:bool)
    n214 = global read "断电保存变量.vi" "pH"() -> (w340:bool)
    n215 = property on="校准选择" class="Clust"() -> ("Controls[]"=w343:refnum<vi>[])  [unwired: 2 in, 2 out]
    n216 = Insert Into Array(array=bool[] [] ("数组"), new element #1=w342, new element #2=w340, new element #3=w339, new element #4=w338, new element #5=w337, new element #6=w336, new element #7=w335, new element #8=w334) -> (w333:bool[])  [unwired: 1 in]
    n217 = for {
      tunnel: w343 -> [w360] mode=indexing
      tunnel: w333 -> [w359] mode=indexing
      n218 = property class="Ctl"(reference=w360, "Visible"=w359) -> ()  [unwired: 1 in, 2 out]
    }
    n219 = property on="藻密度探头选择" class="Ring (严格)"("Visible"=w332) -> ()  [unwired: 2 in, 2 out]
    n220 = property on="DO探头选择" class="Ring (严格)"("Visible"=w332) -> ()  [unwired: 2 in, 2 out]
    n221 = property on="参数设置选项卡" class="TabCtl (严格)"("Visible"=w332) -> ()  [unwired: 2 in, 2 out]
    n222 = property on="浊度探头选择" class="Ring (严格)"("Visible"=w332) -> ()  [unwired: 2 in, 2 out]
    n223 = property on="电导率探头选择" class="Ring (严格)"("Visible"=w332) -> ()  [unwired: 2 in, 2 out]
    n224 = property on="叶绿素a探头选择" class="Ring (严格)"("Visible"=w332) -> ()  [unwired: 2 in, 2 out]
    n225 = property on="ORP探头选择" class="Ring (严格)"("Visible"=w332) -> ()  [unwired: 2 in, 2 out]
    n226 = property on="pH探头选择" class="Ring (严格)"("Visible"=w332) -> ()  [unwired: 2 in, 2 out]
    n227 = property on="自动断线重连" class="Bool (严格)"("Visible"=w350) -> ()  [unwired: 2 in, 2 out]
    n228 = Greater Or Equal?(x=w354, y=u32 1800) -> (x >= y?=w352:bool)
    n229 = local write "密码锁"(w344) -> ()
    n230 = property on="ORP启用" class="Bool (严格)"("DisabledEnum"=w349) -> ()  [unwired: 2 in, 2 out]
    n231 = property on="pH" class="Bool (严格)"("DisabledEnum"=w349) -> ()  [unwired: 2 in, 2 out]
    n232 = property on="DO" class="Bool (严格)"("DisabledEnum"=w349) -> ()  [unwired: 2 in, 2 out]
    n233 = property on="自动断线重连" class="Bool (严格)"("DisabledEnum"=w349) -> ()  [unwired: 2 in, 2 out]
    n234 = property on="Cond" class="Bool (严格)"("DisabledEnum"=w349) -> ()  [unwired: 2 in, 2 out]
    n235 = property on="叶绿素a启用" class="Bool (严格)"("DisabledEnum"=w349) -> ()  [unwired: 2 in, 2 out]
    n236 = property on="Turb" class="Bool (严格)"("DisabledEnum"=w349) -> ()  [unwired: 2 in, 2 out]
    n237 = property on="藻密度" class="Bool (严格)"("DisabledEnum"=w349) -> ()  [unwired: 2 in, 2 out]
    n238 = property on="打开modbus" class="Bool"("DisabledEnum"=w349) -> ()  [unwired: 2 in, 2 out]
    n239 = property on="Temp" class="Bool (严格)"("DisabledEnum"=w349) -> ()  [unwired: 2 in, 2 out]
    n240 = case shown="真" w352 {
      frame False {
      }
      frame True {
        n241 = global write "多参数全局变量.vi" "权限"(enum16{"一级权限", "二级权限", "三级权限"}."一级权限" ("权限")) -> ()
      }
    }
  }
  n242 = while {
    tunnel: w53 -> [w374]
    shift-right: [w373] -> _
    shift-left: u32 0 ("等待时间（毫秒）") -> [w375]
    stop <- FALSE stop-if-true
    # "周期控制"
    n243 = global read "断电保存变量.vi" "定时控制输入"() -> (w377:T15)
    n244 = Wait (ms)(milliseconds to wait=u32 500 ("等待时间（毫秒）")) -> ()  [unwired: 1 out]
    n245 = Unbundle By Name(w377) -> ("周期设置类型"=w379:enum16{"定点启动", "间隔启动"}, "24H周期设置"=w378:bool[], "定时间隔"=w376:u32, "定时功能启用"=w372:bool)
    n246 = case shown="真" w372 {
      tunnel: w379 -> [_ w390]
      tunnel: w378 -> [_ w389]
      tunnel: w376 -> [_ w387]
      tunnel: w375 -> [_ w383]
      tunnel: w374 -> [_ w386]
      tunnel: [_ w382] -> w373
      frame False {
      }
      frame True {
        n247 = property class="VI"(reference=w386) -> ("Exec.State"=w384:T16, "Name"=w385:string)  [unwired: 1 in, 2 out]
        n248 = Get Date/Time In Seconds() -> (seconds since 1Jan1904=w391:timestamp)
        n249 = case shown="\"间隔启动\"" w390 {
          tunnel: w391 -> [w413 _]
          tunnel: w389 -> [w410 _]
          tunnel: [w404 w421] -> w388
          tunnel: w387 -> [_ w420]
          tunnel: w383 -> [_ w422]
          tunnel: [_ w416] -> w382
          frame "定点启动", Default {
            n250 = Seconds To Date/Time(time stamp (now)=w413) -> (date time rec=w412:T17)  [unwired: 1 in]
            n251 = Unbundle By Name(w412) -> ("时"=w411:i32, "分"=w409:i32, "秒"=w408:i32)
            n252 = Index Array(array=w410, index=w411) -> (element=w407:bool)
            n253 = Equal To 0?(x=w409) -> (x = 0?=w406:bool)
            n254 = Equal To 0?(x=w408) -> (x = 0?=w405:bool)
            n255 = Compound Arithmetic op=AND ("复合运算")(w407, w406, w405) -> (w404:bool)
          }
          frame "间隔启动" {
            n256 = Increment(x=w422) -> (x+1=w415:u32)
            n257 = Multiply(x=w420, y=u32 120) -> (x*y=w414:u32)
            n258 = Less?(x=w414, y=w415) -> (x < y?=w418:bool)
            n259 = Select(t=u32 0 ("y"), s=w418, f=w415) -> (s? t:f=w416:u32)
            n260 = Equal To 0?(x=w422) -> (x = 0?=w421:bool)
          }
        }
        n261 = case shown="真" w388 {
          tunnel: w384 -> [_ w393]
          tunnel: w385 -> [_ w392]
          frame False {
          }
          frame True {
            n262 = case shown="\"Idle\"" w393 {
              tunnel: w392 -> [_ w398]
              frame "Bad", Default {
              }
              frame "Idle" {
                n263 = global read "多参数全局变量.vi" "运行模式"() -> (w396:enum16{"维护模式", "常规模式", "应急模式", "质控模式"})
                n264 = case shown="\"常规模式\", 默认" w396 {
                  tunnel: ["M" ("数据标记表") "N" ("数据标记表")] -> w395
                  frame "维护模式" {
                  }
                  frame "常规模式", Default {
                  }
                }
                n265 = Open VI Reference(type specifier VI Refnum (for type only)=refnum<vi> refnum, vi path=w398, options=128 ("选项")) -> (vi reference=w399:refnum<vi>)  [unwired: 3 in, 1 out]
                n266 = call-by-ref "开始异步调用"(reference=w399, "数据标记表"=w395) -> (reference out=w400:refnum<vi>, error out=w401:errorcluster)  [unwired: 12 in]
                n267 = Close Reference(reference=w400, error in (no error)=w401) -> ()  [unwired: 1 out]
              }
            }
          }
        }
      }
    }
    n268 = local write "周期设置"(w372) -> ()
  }
  n269 = property class="VI"(reference=w26) -> ("Library.Version"=w25:T18)  [unwired: 1 in, 2 out]
  n270 = Equal?(x=w10, y="") -> (x = y?=w12:bool)
  n271 = String To IP(1:"192.168.1.100" ("名称")) -> (0:w33:u32)
  n272 = IP To String(1:TRUE ("句点符号？(F)"), 2:w33) -> (0:w30:string)
  n273 = Select(t="1", s=w12, f=w10) -> (s? t:f=w9:string)
  n274 = Unbundle By Name(w25) -> ("Major"=w23:u16, "Minor"=w22:u16, "Fix"=w21:u16, "Build"=w20:u16)
  n275 = call "探头数据读取.vi"("编号"=w9) -> ()  [unwired: 11 in]
  n276 = Concatenate Strings("\\\\" ("字符串"), w30) -> (w31:string)
  n277 = Format Into String(format string="模块版本号：%d.%d.%d.%d" ("格式字符串"), w23, w22, w21, w20) -> (resulting string=→"模块版本号":string)  [unwired: 2 in, 1 out]
  n278 = property class="VI"(reference=w35, error in=errorcluster {"status"=FALSE, "code"=0, "source"=""} ("错误输出")) -> ("Name"=w36:string)  [unwired: 2 out]
  n279 = String To Path(string=w31) -> (path=w28:path)
  n280 = Open VI Reference(type specifier VI Refnum (for type only)=refnum<vi> refnum, vi path=w36, options=128 ("选项")) -> (vi reference=w38:refnum<vi>, error out=w40:errorcluster)  [unwired: 3 in]
  n281 = Build Path(base path=w28, name or relative path=w34) -> (appended path=w4:path)
  n282 = call-by-ref "?"(reference=w38, error in=w40) -> (reference out=w42:refnum<vi>, error out=w41:errorcluster)  [unwired: 12 in]
  n283 = global read "多参数全局变量.vi" "TCP Connection Count"() -> (w5:u32)
  n284 = Close Reference(reference=w42, error in (no error)=w41) -> ()  [unwired: 1 out]
  n285 = case shown="1, 默认" w5 {
    tunnel: w4 -> [w423 w426]
    tunnel: [w423 w425] -> w2
    tunnel: [_ w424] -> w3
    frame 0 {
    }
    frame 1, Default {
      n286 = call <vilib>:"Check if File or Folder Exists.vi"("path"=w426) -> ("file or folder exists?"=w424:bool, "dup path"=w425:path)  [unwired: 8 in, 1 out]
    }
  }
  n287 = case shown="假" w3 {
    tunnel: w2 -> [_ w430]
    tunnel: [w428 w430] -> w7
    tunnel: w34 -> [w427 _]
    frame False {
      # "本地文件地址"
      n288 = call <vilib>:"Application Directory.vi"() -> ("Application Directory"=w429:path)
      n289 = Build Path(base path=w429, name or relative path=w427) -> (appended path=w428:path)
    }
    frame True {
      # "网络共享地址"
    }
  }
  n290 = global write "多参数全局变量.vi" "配置文件 path"(w7) -> ()
  n291 = Equal?(x="编号", y="") -> (x = y?=w17:bool)
  n292 = call <vilib>:"Open Config Data.vi"("configuration file path"=w7) -> ("error out"=w47:errorcluster, "refnum"=w48:T19)  [unwired: 8 in, 1 out]
  n293 = Select(t="1", s=w17, f="编号") -> (s? t:f=w15:string)
  n294 = global write "多参数全局变量.vi" "多参数编号"(w15) -> ()
  n295 = vi-ref "断电保存变量.vi"() -> (w44:refnum<vi>)
  n296 = case shown="\"假\", 默认" w15 {
    tunnel: [TRUE ("可见") FALSE ("可见")] -> w27
    frame "假", Default {
    }
    frame "001" {
    }
  }
  n297 = Concatenate Strings("MPresource" ("名称（未命名）"), w15) -> (w55:string)
  n298 = call <userlib>:"Read Panel from INI__ogtk.vi"("error in (no error)"=w47, "VI ref"=w44, "refnum"=w48) -> ("error out"=w45:errorcluster, "refnum out"=w46:T19)  [unwired: 7 in]
  n299 = Concatenate Strings("MPP" ("名称（未命名）"), w15) -> (w56:string)
  n300 = call <vilib>:"Close Config Data.vi"("error in (no error)"=w45, "refnum"=w46) -> ("error out"=w8:errorcluster)  [unwired: 8 in, 1 out]
  n301 = Obtain Queue(name (unnamed)=w55, element data type="" ("名称（未命名）")) -> (queue out=w51:refnum<queue>)  [unwired: 3 in, 2 out]
  n302 = property on="窗格" class="Pane"("Origin"=T3 {"Horizontal"=0, "Vertical"=0} ("原点")) -> (error out=w63:errorcluster)  [unwired: 2 in, 1 out]
  n303 = Read from Text File(file (use dialog)=w7, error in=w8) -> (error out=w6:errorcluster)  [unwired: 2 in, 3 out]
  n304 = Obtain Notifier(name (unnamed)=w56, notification data type=FALSE) -> (notifier out=w59:refnum<notifier>)  [unwired: 2 in, 2 out]
  n305 = Enqueue Element(queue=w51, element="open" ("元素")) -> (queue out=w50:refnum<queue>)  [unwired: 2 in, 2 out]
  n306 = while {
    tunnel: [w440] -> _
    shift-right: [w433] -> _
    shift-left: _ -> [w438]
    tunnel: w6 -> [w435]
    stop <- FALSE stop-if-true
    n307 = Wait (ms)(milliseconds to wait=u32 1000 ("等待时间（毫秒）")) -> ()  [unwired: 1 out]
    n308 = global read "多参数全局变量.vi" "配置文件 path"() -> (w434:path)
    n309 = File/Directory Info(path=w434, error in=w435) -> (last mod=w433:timestamp, error out=w436:errorcluster)  [unwired: 5 out]
    n310 = Not Equal?(x=w433, y=w438) -> (x != y?=w437:bool)
    n311 = case shown="真" w437 {
      tunnel: [w442 w450] -> w440
      tunnel: w436 -> [w442 w449]
      tunnel: w434 -> [_ w443]
      frame False {
      }
      frame True {
        # "文件发生改变进行更新"
        n312 = call <vilib>:"Open Config Data.vi"("error in (no error)"=w449, "configuration file path"=w443) -> ("error out"=w448:errorcluster, "refnum"=w447:T19)  [unwired: 7 in, 1 out]
        n313 = vi-ref "断电保存变量.vi"() -> (w444:refnum<vi>)
        n314 = call <userlib>:"Read Panel from INI__ogtk.vi"("error in (no error)"=w448, "VI ref"=w444, "refnum"=w447) -> ("error out"=w446:errorcluster, "refnum out"=w445:T19)  [unwired: 7 in]
        n315 = call <vilib>:"Close Config Data.vi"("error in (no error)"=w446, "refnum"=w445) -> ("error out"=w450:errorcluster)  [unwired: 8 in, 1 out]
      }
    }
  }
  n316 = while {
    tunnel: w50 -> [w452]
    tunnel: w6 -> [_]
    stop <- FALSE stop-if-true
    n317 = Dequeue Element(queue=w452) -> (element=w451:string)  [unwired: 2 in, 3 out]
    n318 = case shown="\"open\"" w451 {
      tunnel: [_ w454 w464] -> _
      frame "假", Default {
      }
      frame "open" {
        n319 = global read "多参数全局变量.vi" "MB session in"() -> (w459:refnum<class "MB_Master.lvclass">)
        n320 = global read "断电保存变量.vi" "VISA资源名称"() -> (w461:refnum<visa-resource-name>)
        n321 = global read "断电保存变量.vi" "连接方式"() -> (w457:u16)
        n322 = call "close MB.vi"("MB session in"=w459) -> ("error out"=w462:errorcluster)  [unwired: 10 in]
        n323 = global read "断电保存变量.vi" "Port"() -> (w455:u16)
        n324 = global read "断电保存变量.vi" "IP"() -> (w456:string)
        n325 = call "open MB.vi"("Port (502)"=w455, "IP Address"=w456, "MODE"=w457, "error in (no error)"=w462, "Serial Config"=T20 {"baud rate (bps)"=9600, "stop bits"=10, "parity"=0, "flow control"=0, "timeout"=1000, "retries"=1}, "VISA资源名称"=w461) -> ("error out"=w454:errorcluster, "MB session out"=w458:refnum<class "MB_Master.lvclass">)  [unwired: 4 in]
        n326 = global write "多参数全局变量.vi" "MB session in"(w458) -> ()
      }
      frame "close" {
        n327 = global read "多参数全局变量.vi" "MB session in"() -> (w463:refnum<class "MB_Master.lvclass">)
        n328 = call "close MB.vi"("MB session in"=w463) -> ("error out"=w464:errorcluster)  [unwired: 10 in]
      }
    }
  }
  n329 = while {
    tunnel: w50 -> [w466]
    stop <- FALSE stop-if-true
    # "断线重连"
    n330 = global read "断电保存变量.vi" "连接方式"() -> (w467:u16)
    n331 = Wait (ms)(milliseconds to wait=u32 10000 ("等待时间（毫秒）")) -> ()  [unwired: 1 out]
    n332 = case shown="1" w467 {
      tunnel: w466 -> [_ w470]
      frame 0, Default {
      }
      frame 1 {
        n333 = case shown="真" "自动断线重连" {
          tunnel: w470 -> [_ w473]
          frame False {
          }
          frame True {
            n334 = global read "多参数全局变量.vi" "MB session in"() -> (w472:refnum<class "MB_Master.lvclass">)
            n335 = property class="MB_Master"(reference=w472) -> ("Properties:Session Valid"=w471:bool)  [unwired: 1 in, 2 out]
            n336 = case shown="假" w471 {
              tunnel: w473 -> [w474 _]
              frame False {
                n337 = Flush Queue(queue=w474) -> (queue out=w476:refnum<queue>)  [unwired: 1 in, 2 out]
                n338 = Enqueue Element(queue=w476, element="open" ("元素")) -> ()  [unwired: 2 in, 3 out]
              }
              frame True {
              }
            }
          }
        }
      }
    }
  }
  n339 = while {
    tunnel: w63 -> [_]
    tunnel: w59 -> [w478]
    tunnel: w50 -> [w477]
    stop <- FALSE stop-if-true
    n340 = event shown="[12] \"仪器参数\": 值改变" {
      selector: _ -> [_ _ _ _ _ _ _ _ _ _ _ _ _ _ _ _ _ _ _ _ _ _ _ _]
      dyn-events: _ -> [_ _ _ _ _ _ _ _ _ _ _ _ _ _ _ _ _ _ _ _ _ _ _ _]
      timeout: _ -> [_ _ _ _ _ _ _ _ _ _ _ _ _ _ _ _ _ _ _ _ _ _ _ _]
      tunnel: w478 -> [_ _ _ _ _ _ _ _ _ _ w580 _ _ _ _ _ _ _ _ _ _ _ _ _]
      tunnel: w477 -> [_ _ _ _ _ _ _ _ _ _ _ _ _ _ w618 _ _ _ _ _ _ _ _ _]
      event Timeout {
        n341 = event-data() -> ()  [unwired: 1 in, 3 out]
      }
      event "水样测量时间": Mouse Down {
        n342 = event-data() -> ("CtlRef"=w480:refnum<vi>)  [unwired: 1 in, 5 out]
        n343 = property class="DigNum (严格)"(reference=w480) -> (reference out=w483:refnum<vi>, "Value"=w482:dbl)  [unwired: 1 in, 1 out]
        n344 = call "数字键盘.vi"("OldNumber"=w482) -> ("NewNumber"=w481:dbl)  [unwired: 1 in]
        n345 = property class="DigNum (严格)"(reference=w483, "Val(Sgnl)"=w481) -> ()  [unwired: 1 in, 2 out]
      }
      event "pH探头选择", "DO探头选择", "电导率探头选择", "浊度探头选择", "叶绿素a探头选择", "藻密度探头选择", "ORP探头选择": Value Change {
        n346 = event-data() -> ("CtlRef"=w484:refnum<vi>, "NewVal"=w485:u16)  [unwired: 1 in, 4 out]
        n347 = Two Button Dialog(message="请再次确认修改的型号是否与实际匹配，否则将导致通讯异常，并且此操作将终止所有正在校准的参数！" ("消息")) -> (T button?=w486:bool)  [unwired: 2 in]
        n348 = case shown="真" w486 {
          tunnel: w485 -> [_ w489]
          tunnel: w484 -> [_ w488]
          frame False {
          }
          frame True {
            n349 = flat-sequence {
              tunnel: w489 -> [w490]
              tunnel: w488 -> [w494]
              frame #0 {
                n350 = property class="Ring (严格)"(reference=w494) -> ("Label.Text"=w493:string)  [unwired: 1 in, 2 out]
                n351 = global read "断电保存变量.vi" "探头选择"() -> (w492:T13)
                n352 = global read "多参数全局变量.vi" "校准VI引用句柄"() -> (w495:T21)
                n353 = case shown="\"ORP探头选择\"" w493 {
                  tunnel: w492 -> [w497 w500 w503 w506 w509 w512 w515 w518]
                  tunnel: [w497 w499 w502 w505 w508 w511 w514 w517] -> w491
                  tunnel: w490 -> [_ w498 w501 w504 w507 w510 w513 w516]
                  frame Default {
                  }
                  frame "pH探头选择" {
                    n354 = Bundle By Name(cluster=w500, "pH探头选择"=w498) -> (w499:T13)
                  }
                  frame "电导率探头选择" {
                    n355 = Bundle By Name(cluster=w503, "电导率探头选择"=w501) -> (w502:T13)
                  }
                  frame "DO探头选择" {
                    n356 = Bundle By Name(cluster=w506, "DO探头选择"=w504) -> (w505:T13)
                  }
                  frame "浊度探头选择" {
                    n357 = Bundle By Name(cluster=w509, "浊度探头选择"=w507) -> (w508:T13)
                  }
                  frame "叶绿素a探头选择" {
                    n358 = Bundle By Name(cluster=w512, "叶绿素a探头选择"=w510) -> (w511:T13)
                  }
                  frame "蓝绿藻探头选择" {
                    n359 = Bundle By Name(cluster=w515, "蓝绿藻探头选择"=w513) -> (w514:T13)
                  }
                  frame "ORP探头选择" {
                    n360 = Bundle By Name(cluster=w518, "蓝绿藻探头选择"=w516) -> (w517:T13)
                  }
                }
                n361 = Cluster To Array(cluster=w495) -> (array=w496:refnum<vi>[])
                n362 = for {
                  tunnel: w496 -> [w520] mode=indexing
                  tunnel: [w519] -> _ mode=indexing
                  n363 = invoke class="VI" method="Abort VI"(reference=w520) -> (error out=w519:errorcluster)  [unwired: 2 in, 2 out]
                }
                n364 = global write "断电保存变量.vi" "探头选择"(w491) -> ()
              }
              frame #1 {
                n365 = call "配置文件保存.vi"() -> ()  [unwired: 12 in]
              }
            }
          }
        }
      }
      event "VISA资源名称", "pH", "DO", "Turb", "Cond", "Temp", "叶绿素a启用", "打开modbus", "藻密度", "连接方式", "自动断线重连", "ORP启用": Mouse Down {
        n366 = event-data() -> ()  [unwired: 1 in, 6 out]
        n367 = local read "密码锁"() -> (w521:bool)
        n368 = case shown="假" w521 {
          frame False {
            n369 = One Button Dialog(message="当前操作权限不足,请提升权限!!!" ("消息")) -> ()  [unwired: 1 in, 1 out]
          }
          frame True {
          }
        }
      }
      event "IP": Mouse Down {
        n370 = event-data() -> ("CtlRef"=w524:refnum<vi>)  [unwired: 1 in, 7 out]
        n371 = property on="IP" class="Str"() -> ("DisabledEnum"=w523:T12)  [unwired: 2 in, 2 out]
        n372 = case shown="\"Disabled and Grayed Out\"" w523 {
          tunnel: w524 -> [w528 _ _]
          frame "Enabled" {
            n373 = property class="Str"(reference=w528) -> (reference out=w527:refnum<vi>, "Value"=w526:string)  [unwired: 1 in, 1 out]
            n374 = call "字符键盘.vi"("Old String"=w526) -> ("String"=w525:string)  [unwired: 10 in]
            n375 = property class="Str"(reference=w527, "Val(Sgnl)"=w525) -> ()  [unwired: 1 in, 2 out]
          }
          frame "Disabled and Grayed Out" {
            n376 = One Button Dialog(message="关闭连接后才可设置!" ("消息")) -> ()  [unwired: 1 in, 1 out]
          }
          frame "Disabled", Default {
            n377 = One Button Dialog(message="当前操作权限不足,请提升权限!!!" ("消息")) -> ()  [unwired: 1 in, 1 out]
          }
        }
      }
      event "Port": Mouse Down {
        n378 = event-data() -> ("CtlRef"=w532:refnum<vi>)  [unwired: 1 in, 7 out]
        n379 = property on="Port" class="DigNum (严格)"() -> ("DisabledEnum"=w531:T12)  [unwired: 2 in, 2 out]
        n380 = case shown="\"Enabled\"" w531 {
          tunnel: w532 -> [w536 _ _]
          frame "Enabled" {
            n381 = property class="DigNum (严格)"(reference=w536) -> (reference out=w535:refnum<vi>, "Value"=w534:u16)  [unwired: 1 in, 1 out]
            n382 = call "数字键盘.vi"("OldNumber"=w534) -> ("NewNumber"=w533:dbl)  [unwired: 1 in]
            n383 = property class="DigNum (严格)"(reference=w535, "Val(Sgnl)"=w533) -> ()  [unwired: 1 in, 2 out]
          }
          frame "Disabled and Grayed Out" {
            n384 = One Button Dialog(message="关闭连接后才可设置!" ("消息")) -> ()  [unwired: 1 in, 1 out]
          }
          frame "Disabled", Default {
            n385 = One Button Dialog(message="当前操作权限不足,请提升权限!!!" ("消息")) -> ()  [unwired: 1 in, 1 out]
          }
        }
      }
      event "密码锁": Value Change {
        n386 = event-data() -> ("NewVal"=w539:bool)  [unwired: 1 in, 5 out]
        n387 = case shown="假" w539 {
          frame False {
            n388 = global write "多参数全局变量.vi" "权限"(enum16{"一级权限", "二级权限", "三级权限"}."一级权限" ("权限")) -> ()
          }
          frame True {
            n389 = call "数字键盘.vi"("显示样式"=u32 2) -> ("NewNumber"=w544:dbl)  [unwired: 1 in]
            n390 = case shown="23506" w544 {
              tunnel: ["密码错误,即将切换为一级权限!" ("Infoin") "密码正确,即将切换为二级权限!" ("Infoin") "密码正确,即将切换为三级权限!" ("Infoin")] -> w543
              tunnel: [u32 16711680 ("颜色盒") _ _] -> w542
              tunnel: [enum16{"一级权限", "二级权限", "三级权限"}."一级权限" ("权限") enum16{"一级权限", "二级权限", "三级权限"}."二级权限" ("权限") enum16{"一级权限", "二级权限", "三级权限"}."三级权限" ("权限")] -> w541
              frame 0, Default {
              }
              frame 666 {
              }
              frame 23506 {
              }
            }
            n391 = global write "多参数全局变量.vi" "权限"(w541) -> ()
            n392 = call "TimeLmtDialog.vi"("颜色盒"=w542, "Infoin"=w543) -> ()  [unwired: 10 in]
          }
        }
      }
      event "周期设置": Mouse Down {
        n393 = event-data() -> ()  [unwired: 1 in, 6 out]
        n394 = flat-sequence {
          frame #0 {
            n395 = global read "断电保存变量.vi" "定时控制输入"() -> (w554:T15)
            n396 = call "周期设置.vi"("定时控制输入"=w554) -> ("定时控制输出"=w553:T15)  [unwired: 10 in]
            n397 = global write "断电保存变量.vi" "定时控制输入"(w553) -> ()
          }
          frame #1 {
            n398 = call "配置文件保存.vi"() -> ()  [unwired: 12 in]
          }
        }
      }
      event "水样测试": Value Change {
        n399 = event-data() -> ()  [unwired: 1 in, 6 out]
        n400 = vi-ref "水样测试.vi"() -> (w557:refnum<vi>)
        n401 = property class="VI"(reference=w557) -> ("Name"=w561:string, "Exec.State"=w559:T16)  [unwired: 1 in, 2 out]
        n402 = Open VI Reference(type specifier VI Refnum (for type only)=refnum<vi> refnum, vi path=w561, options=128 ("选项")) -> (vi reference=w562:refnum<vi>)  [unwired: 3 in, 1 out]
        n403 = case shown="\"Idle\"" w559 {
          tunnel: [w563 w566] -> w558
          tunnel: w562 -> [w563 w565]
          tunnel: "hd" ("数据标记表") -> [_ w564]
          frame "Bad", Default {
          }
          frame "Idle" {
            n404 = call-by-ref "开始异步调用"(reference=w565, "数据标记表"=w564) -> (reference out=w566:refnum<vi>)  [unwired: 12 in, 1 out]
          }
        }
        n405 = Close Reference(reference=w558) -> ()  [unwired: 1 in, 1 out]
      }
      event "标样核查": Value Change {
        n406 = event-data() -> ()  [unwired: 1 in, 6 out]
        n407 = call "标样核查配置.vi"() -> ("确认输出"=w567:bool)  [unwired: 11 in]
        n408 = case shown="真" w567 {
          frame False {
          }
          frame True {
            n409 = vi-ref "标样核查.vi"() -> (w569:refnum<vi>)
            n410 = property class="VI"(reference=w569) -> ("Name"=w573:string, "Exec.State"=w571:T16)  [unwired: 1 in, 2 out]
            n411 = Open VI Reference(type specifier VI Refnum (for type only)=refnum<vi> refnum, vi path=w573, options=128 ("选项")) -> (vi reference=w574:refnum<vi>)  [unwired: 3 in, 1 out]
            n412 = case shown="\"Idle\"" w571 {
              tunnel: [w575 w577] -> w570
              tunnel: w574 -> [w575 w576]
              frame "Bad", Default {
              }
              frame "Idle" {
                n413 = call-by-ref "开始异步调用"(reference=w576) -> (reference out=w577:refnum<vi>)  [unwired: 13 in, 1 out]
              }
            }
            n414 = Close Reference(reference=w570) -> ()  [unwired: 1 in, 1 out]
          }
        }
      }
      event "停止": Value Change {
        w578 = u16 3 items=["空闲", "水样测试", "标样核查", "停止"] ("主副屏同步启动")
        n415 = event-data() -> ()  [unwired: 1 in, 6 out]
        n416 = Send Notification(notification=TRUE ("通知"), notifier=w580) -> ()  [unwired: 1 in, 2 out]
        n417 = global write "多参数全局变量.vi" "主副屏同步启动"(w578) -> ()
      }
      event "设置": Value Change {
        n418 = event-data() -> ()  [unwired: 1 in, 6 out]
        n419 = property on="窗格" class="Pane"("Origin"=T3 {"Horizontal"=0, "Vertical"=628} ("原点")) -> ()  [unwired: 2 in, 2 out]
      }
      event "仪器参数": Value Change {
        n420 = event-data() -> ()  [unwired: 1 in, 6 out]
        n421 = global read "断电保存变量.vi" "叶绿素参数"() -> (w582:T10)
        n422 = global read "断电保存变量.vi" "藻密度参数"() -> (w583:T10)
        n423 = global read "断电保存变量.vi" "电导率参数"() -> (w590:T10)
        n424 = global read "断电保存变量.vi" "溶解氧参数"() -> (w588:T10)
        n425 = global read "断电保存变量.vi" "ORP参数"() -> (w584:T10)
        n426 = global read "断电保存变量.vi" "水温参数"() -> (w591:T10)
        n427 = global read "断电保存变量.vi" "浊度参数"() -> (w589:T10)
        n428 = global read "断电保存变量.vi" "PH参数"() -> (w592:T10)
        n429 = Build Array(w592, w591, w590, w588, w589, w582, w583, w584) -> (w587:T22)
        n430 = call "仪器参数设置.vi"("仪器参数设置输入"=w587) -> ("确定"=w586:bool, "仪器参数设置输出"=w585:T22)  [unwired: 9 in]
        n431 = case shown="真" w586 {
          tunnel: w585 -> [_ w593]
          frame False {
          }
          frame True {
            n432 = flat-sequence {
              tunnel: w593 -> [w602]
              frame #0 {
                n433 = Index Array(array=w602) -> (element #1=w600:T10, element #2=w599:T10, element #3=w597:T10, element #4=w598:T10, element #5=w601:T10, element #6=w596:T10, element #7=w594:T10, element #8=w595:T10)  [unwired: 8 in]
                n434 = global write "断电保存变量.vi" "叶绿素参数"(w596) -> ()
                n435 = global write "断电保存变量.vi" "藻密度参数"(w594) -> ()
                n436 = global write "断电保存变量.vi" "PH参数"(w600) -> ()
                n437 = global write "断电保存变量.vi" "水温参数"(w599) -> ()
                n438 = global write "断电保存变量.vi" "电导率参数"(w597) -> ()
                n439 = global write "断电保存变量.vi" "溶解氧参数"(w598) -> ()
                n440 = global write "断电保存变量.vi" "浊度参数"(w601) -> ()
                n441 = global write "断电保存变量.vi" "ORP参数"(w595) -> ()
              }
              frame #1 {
                n442 = call "配置文件保存.vi"() -> ()  [unwired: 12 in]
              }
            }
          }
        }
      }
      event "pH", "DO", "Turb", "Cond", "Temp", "叶绿素a启用", "藻密度", "VISA资源名称", "连接方式", "IP", "Port", "自动断线重连", "水样测量时间", "ORP启用": Value Change {
        n443 = event-data() -> ()  [unwired: 1 in, 6 out]
        n444 = flat-sequence {
          frame #0 {
            n445 = global write "断电保存变量.vi" "IP"("IP") -> ()
            n446 = global write "断电保存变量.vi" "藻密度"("藻密度") -> ()
            n447 = global write "断电保存变量.vi" "连接方式"("连接方式") -> ()
            n448 = global write "断电保存变量.vi" "Temp"("Temp") -> ()
            n449 = global write "断电保存变量.vi" "DO"("DO") -> ()
            n450 = global write "断电保存变量.vi" "Turb"("Turb") -> ()
            n451 = global write "断电保存变量.vi" "Port"("Port") -> ()
            n452 = global write "断电保存变量.vi" "pH"("pH") -> ()
            n453 = global write "断电保存变量.vi" "orp"("ORP启用") -> ()
            n454 = global write "断电保存变量.vi" "Cond"("Cond") -> ()
            n455 = global write "断电保存变量.vi" "叶绿素a启用"("叶绿素a启用") -> ()
            n456 = global write "断电保存变量.vi" "VISA资源名称"("VISA资源名称") -> ()
            n457 = global write "断电保存变量.vi" "水样测定时间"("水样测量时间") -> ()
            n458 = local read "自动断线重连"() -> (w605:bool)
            n459 = global write "断电保存变量.vi" "自动断线重连"(w605) -> ()
          }
          frame #1 {
            n460 = call "配置文件保存.vi"() -> ()  [unwired: 12 in]
          }
          frame #2 {
          }
        }
      }
      event "打开modbus": Value Change {
        n461 = event-data() -> ()  [unwired: 1 in, 6 out]
        n462 = global read "多参数全局变量.vi" "MB session in"() -> (w623:refnum<class "MB_Master.lvclass">)
        n463 = Flush Queue(queue=w618) -> (queue out=w617:refnum<queue>)  [unwired: 1 in, 2 out]
        n464 = property class="MB_Master"(reference=w623) -> ("Properties:Session Valid"=w622:bool)  [unwired: 1 in, 2 out]
        n465 = Select(t="close" ("元素"), s=w622, f="open" ("元素")) -> (s? t:f=w619:string)
        n466 = Enqueue Element(queue=w617, element=w619) -> ()  [unwired: 2 in, 3 out]
      }
      event "探头校正返回", "设置页返回": Value Change {
        n467 = event-data() -> ()  [unwired: 1 in, 6 out]
        n468 = property on="窗格" class="Pane"("Origin"=T3 {"Horizontal"=0, "Vertical"=0} ("原点")) -> ()  [unwired: 2 in, 2 out]
      }
      event "探头校正", "校准选择.水温校准": Value Change {
        n469 = event-data() -> ()  [unwired: 1 in, 6 out]
        n470 = property on="窗格" class="Pane"("Origin"=T3 {"Horizontal"=1656, "Vertical"=0} ("原点")) -> ()  [unwired: 2 in, 2 out]
        n471 = vi-ref "水温校准.vi"() -> (w625:refnum<vi>)
        n472 = property class="VI"(reference=w625) -> (reference out=w627:refnum<vi>, "Exec.State"=w626:T16)  [unwired: 1 in, 1 out]
        n473 = case shown="\"Bad\", 默认" w626 {
          tunnel: [w631 w633] -> w629
          tunnel: w627 -> [w631 w632]
          frame "Bad", Default {
          }
          frame "Idle" {
            n474 = invoke class="VI" method="Run VI"(reference=w632, "Wait until done"=FALSE ("结束前等待"), "Auto Dispose Ref"=FALSE ("自动销毁引用")) -> (reference out=w633:refnum<vi>)  [unwired: 2 in, 4 out]
          }
        }
        n475 = invoke on="探头校准子面板" class="SubPnl" method="Remove VI"() -> (error out=w628:errorcluster)  [unwired: 3 in, 2 out]
        n476 = invoke on="探头校准子面板" class="SubPnl" method="Insert VI"(error in=w628, "VI Ref"=w629) -> ()  [unwired: 2 in, 4 out]
      }
      event "校准选择.pH校准": Value Change {
        n477 = event-data() -> ()  [unwired: 1 in, 6 out]
        n478 = global read "断电保存变量.vi" "探头选择"() -> (w641:T13)
        n479 = Unbundle By Name(w641) -> ("pH探头选择"=w640:u16)
        n480 = case shown="2" w640 {
          tunnel: [w645 w646 w647] -> w639
          frame 0, Default {
            n481 = vi-ref "斯坦道多参数.lvlib:禹山pH校准.vi"() -> (w645:refnum<vi>)
          }
          frame 1 {
            n482 = vi-ref "斯坦道多参数.lvlib:pH电极校准.vi"() -> (w646:refnum<vi>)
          }
          frame 2 {
            n483 = vi-ref "斯坦道多参数.lvlib:纳清pH电极校准.vi"() -> (w647:refnum<vi>)
          }
        }
        n484 = property class="VI"(reference=w639) -> (reference out=w643:refnum<vi>, "Exec.State"=w642:T16)  [unwired: 1 in, 1 out]
        n485 = case shown="\"Bad\", 默认" w642 {
          tunnel: w643 -> [w648 w652]
          tunnel: [w648 w649] -> w637
          frame "Bad", Default {
          }
          frame "Idle" {
            n486 = invoke class="VI" method="Run VI"(reference=w652, "Wait until done"=FALSE ("结束前等待"), "Auto Dispose Ref"=FALSE ("自动销毁引用")) -> (reference out=w649:refnum<vi>)  [unwired: 2 in, 4 out]
          }
        }
        n487 = global read "多参数全局变量.vi" "校准VI引用句柄"() -> (w638:T21)
        n488 = invoke on="探头校准子面板" class="SubPnl" method="Remove VI"() -> (error out=w644:errorcluster)  [unwired: 3 in, 2 out]
        n489 = invoke on="探头校准子面板" class="SubPnl" method="Insert VI"(error in=w644, "VI Ref"=w637) -> ()  [unwired: 2 in, 4 out]
        n490 = Bundle By Name(cluster=w638, "pH校准VI引用句柄"=w637) -> (w636:T21)
        n491 = global write "多参数全局变量.vi" "校准VI引用句柄"(w636) -> ()
      }
      event "校准选择.电导率校准": Value Change {
        n492 = event-data() -> ()  [unwired: 1 in, 6 out]
        n493 = global read "断电保存变量.vi" "探头选择"() -> (w658:T13)
        n494 = Unbundle By Name(w658) -> ("电导率探头选择"=w657:u16)
        n495 = case shown="2" w657 {
          tunnel: [w662 w663 w664] -> w656
          frame 0, Default {
            n496 = vi-ref "斯坦道多参数.lvlib:禹山电导率校准.vi"() -> (w662:refnum<vi>)
          }
          frame 1 {
            n497 = vi-ref "斯坦道多参数.lvlib:电导率电极校准.vi"() -> (w663:refnum<vi>)
          }
          frame 2 {
            n498 = vi-ref "斯坦道多参数.lvlib:纳清电导率电极校准.vi"() -> (w664:refnum<vi>)
          }
        }
        n499 = property class="VI"(reference=w656) -> (reference out=w660:refnum<vi>, "Exec.State"=w659:T16)  [unwired: 1 in, 1 out]
        n500 = case shown="\"Bad\", 默认" w659 {
          tunnel: [w665 w667] -> w653
          tunnel: w660 -> [w665 w666]
          frame "Bad", Default {
          }
          frame "Idle" {
            n501 = invoke class="VI" method="Run VI"(reference=w666, "Wait until done"=FALSE ("结束前等待"), "Auto Dispose Ref"=FALSE ("自动销毁引用")) -> (reference out=w667:refnum<vi>)  [unwired: 2 in, 4 out]
          }
        }
        n502 = global read "多参数全局变量.vi" "校准VI引用句柄"() -> (w655:T21)
        n503 = invoke on="探头校准子面板" class="SubPnl" method="Remove VI"() -> (error out=w661:errorcluster)  [unwired: 3 in, 2 out]
        n504 = Bundle By Name(cluster=w655, "COND校准VI引用句柄"=w653) -> (w654:T21)
        n505 = invoke on="探头校准子面板" class="SubPnl" method="Insert VI"(error in=w661, "VI Ref"=w653) -> ()  [unwired: 2 in, 4 out]
        n506 = global write "多参数全局变量.vi" "校准VI引用句柄"(w654) -> ()
      }
      event "校准选择.溶解氧校准": Value Change {
        n507 = event-data() -> ()  [unwired: 1 in, 6 out]
        n508 = global read "断电保存变量.vi" "探头选择"() -> (w675:T13)
        n509 = Unbundle By Name(w675) -> ("DO探头选择"=w674:u16)
        n510 = case shown="2" w674 {
          tunnel: [w679 w680 w681] -> w673
          frame 0, Default {
            n511 = vi-ref "斯坦道多参数.lvlib:禹山溶解氧校准.vi"() -> (w679:refnum<vi>)
          }
          frame 1 {
            n512 = vi-ref "斯坦道多参数.lvlib:溶解氧电极校准.vi"() -> (w680:refnum<vi>)
          }
          frame 2 {
            n513 = vi-ref "斯坦道多参数.lvlib:纳清DO电极校准.vi"() -> (w681:refnum<vi>)
          }
        }
        n514 = property class="VI"(reference=w673) -> (reference out=w677:refnum<vi>, "Exec.State"=w676:T16)  [unwired: 1 in, 1 out]
        n515 = case shown="\"Bad\", 默认" w676 {
          tunnel: [w682 w684] -> w670
          tunnel: w677 -> [w682 w683]
          frame "Bad", Default {
          }
          frame "Idle" {
            n516 = invoke class="VI" method="Run VI"(reference=w683, "Wait until done"=FALSE ("结束前等待"), "Auto Dispose Ref"=FALSE ("自动销毁引用")) -> (reference out=w684:refnum<vi>)  [unwired: 2 in, 4 out]
          }
        }
        n517 = global read "多参数全局变量.vi" "校准VI引用句柄"() -> (w672:T21)
        n518 = invoke on="探头校准子面板" class="SubPnl" method="Remove VI"() -> (error out=w678:errorcluster)  [unwired: 3 in, 2 out]
        n519 = invoke on="探头校准子面板" class="SubPnl" method="Insert VI"(error in=w678, "VI Ref"=w670) -> ()  [unwired: 2 in, 4 out]
        n520 = Bundle By Name(cluster=w672, "DO校准VI引用句柄"=w670) -> (w671:T21)
        n521 = global write "多参数全局变量.vi" "校准VI引用句柄"(w671) -> ()
      }
      event "校准选择.浊度校准": Value Change {
        n522 = event-data() -> ()  [unwired: 1 in, 6 out]
        n523 = global read "断电保存变量.vi" "探头选择"() -> (w692:T13)
        n524 = Unbundle By Name(w692) -> ("浊度探头选择"=w691:u16)
        n525 = case shown="2" w691 {
          tunnel: [w696 w697 w698] -> w690
          frame 0, Default {
            n526 = vi-ref "斯坦道多参数.lvlib:禹山浊度校准.vi"() -> (w696:refnum<vi>)
          }
          frame 1 {
            n527 = vi-ref "斯坦道多参数.lvlib:浊度电极校准.vi"() -> (w697:refnum<vi>)
          }
          frame 2 {
            n528 = vi-ref "斯坦道多参数.lvlib:纳清浊度电极校准.vi"() -> (w698:refnum<vi>)
          }
        }
        n529 = property class="VI"(reference=w690) -> (reference out=w694:refnum<vi>, "Exec.State"=w693:T16)  [unwired: 1 in, 1 out]
        n530 = case shown="\"Bad\", 默认" w693 {
          tunnel: [w699 w701] -> w687
          tunnel: w694 -> [w699 w700]
          frame "Bad", Default {
          }
          frame "Idle" {
            n531 = invoke class="VI" method="Run VI"(reference=w700, "Wait until done"=FALSE ("结束前等待"), "Auto Dispose Ref"=FALSE ("自动销毁引用")) -> (reference out=w701:refnum<vi>)  [unwired: 2 in, 4 out]
          }
        }
        n532 = global read "多参数全局变量.vi" "校准VI引用句柄"() -> (w689:T21)
        n533 = invoke on="探头校准子面板" class="SubPnl" method="Remove VI"() -> (error out=w695:errorcluster)  [unwired: 3 in, 2 out]
        n534 = invoke on="探头校准子面板" class="SubPnl" method="Insert VI"(error in=w695, "VI Ref"=w687) -> ()  [unwired: 2 in, 4 out]
        n535 = Bundle By Name(cluster=w689, "TURB校准VI引用句柄"=w687) -> (w688:T21)
        n536 = global write "多参数全局变量.vi" "校准VI引用句柄"(w688) -> ()
      }
      event "校准选择.叶绿素a校准": Value Change {
        n537 = event-data() -> ()  [unwired: 1 in, 6 out]
        n538 = global read "断电保存变量.vi" "探头选择"() -> (w708:T13)
        n539 = Unbundle By Name(w708) -> ("叶绿素a探头选择"=w707:u16)
        n540 = case shown="2" w707 {
          tunnel: [w713 _ w714] -> w709
          frame 0, Default {
            n541 = vi-ref "禹山叶绿素a校准.vi"() -> (w713:refnum<vi>)
          }
          frame 1 {
          }
          frame 2 {
            n542 = vi-ref "斯坦道多参数.lvlib:纳清叶绿素a电极校准.vi"() -> (w714:refnum<vi>)
          }
        }
        n543 = property class="VI"(reference=w709) -> (reference out=w711:refnum<vi>, "Exec.State"=w710:T16)  [unwired: 1 in, 1 out]
        n544 = case shown="\"Bad\", 默认" w710 {
          tunnel: [w715 w717] -> w704
          tunnel: w711 -> [w715 w716]
          frame "Bad", Default {
          }
          frame "Idle" {
            n545 = invoke class="VI" method="Run VI"(reference=w716, "Wait until done"=FALSE ("结束前等待"), "Auto Dispose Ref"=FALSE ("自动销毁引用")) -> (reference out=w717:refnum<vi>)  [unwired: 2 in, 4 out]
          }
        }
        n546 = global read "多参数全局变量.vi" "校准VI引用句柄"() -> (w706:T21)
        n547 = invoke on="探头校准子面板" class="SubPnl" method="Remove VI"() -> (error out=w712:errorcluster)  [unwired: 3 in, 2 out]
        n548 = invoke on="探头校准子面板" class="SubPnl" method="Insert VI"(error in=w712, "VI Ref"=w704) -> ()  [unwired: 2 in, 4 out]
        n549 = Bundle By Name(cluster=w706, "CHLA校准VI引用句柄"=w704) -> (w705:T21)
        n550 = global write "多参数全局变量.vi" "校准VI引用句柄"(w705) -> ()
      }
      event "校准选择.藻密度校准": Value Change {
        n551 = event-data() -> ()  [unwired: 1 in, 6 out]
        n552 = global read "断电保存变量.vi" "探头选择"() -> (w724:T13)
        n553 = Unbundle By Name(w724) -> ("蓝绿藻探头选择"=w723:u16)
        n554 = case shown="2" w723 {
          tunnel: [_ w729] -> w725
          frame 0, Default {
          }
          frame 2 {
            n555 = vi-ref "斯坦道多参数.lvlib:纳清蓝绿藻电极校准.vi"() -> (w729:refnum<vi>)
          }
        }
        n556 = property class="VI"(reference=w725) -> (reference out=w727:refnum<vi>, "Exec.State"=w726:T16)  [unwired: 1 in, 1 out]
        n557 = case shown="\"Bad\", 默认" w726 {
          tunnel: [w730 w732] -> w720
          tunnel: w727 -> [w730 w731]
          frame "Bad", Default {
          }
          frame "Idle" {
            n558 = invoke class="VI" method="Run VI"(reference=w731, "Wait until done"=FALSE ("结束前等待"), "Auto Dispose Ref"=FALSE ("自动销毁引用")) -> (reference out=w732:refnum<vi>)  [unwired: 2 in, 4 out]
          }
        }
        n559 = global read "多参数全局变量.vi" "校准VI引用句柄"() -> (w722:T21)
        n560 = invoke on="探头校准子面板" class="SubPnl" method="Remove VI"() -> (error out=w728:errorcluster)  [unwired: 3 in, 2 out]
        n561 = invoke on="探头校准子面板" class="SubPnl" method="Insert VI"(error in=w728, "VI Ref"=w720) -> ()  [unwired: 2 in, 4 out]
        n562 = Bundle By Name(cluster=w722, "BGA校准VI引用句柄"=w720) -> (w721:T21)
        n563 = global write "多参数全局变量.vi" "校准VI引用句柄"(w721) -> ()
      }
      event "校准选择.ORP校准": Value Change {
        n564 = event-data() -> ()  [unwired: 1 in, 6 out]
        n565 = global read "断电保存变量.vi" "探头选择"() -> (w739:T13)
        n566 = Unbundle By Name(w739) -> ("orp探头选择"=w738:u16)
        n567 = case shown="1" w738 {
          tunnel: [_ w744] -> w740
          frame 0, Default {
          }
          frame 1 {
            n568 = vi-ref "斯坦道多参数.lvlib:ORP电极校准.vi"() -> (w744:refnum<vi>)
          }
        }
        n569 = property class="VI"(reference=w740) -> (reference out=w742:refnum<vi>, "Exec.State"=w741:T16)  [unwired: 1 in, 1 out]
        n570 = case shown="\"Bad\", 默认" w741 {
          tunnel: [w745 w747] -> w735
          tunnel: w742 -> [w745 w746]
          frame "Bad", Default {
          }
          frame "Idle" {
            n571 = invoke class="VI" method="Run VI"(reference=w746, "Wait until done"=FALSE ("结束前等待"), "Auto Dispose Ref"=FALSE ("自动销毁引用")) -> (reference out=w747:refnum<vi>)  [unwired: 2 in, 4 out]
          }
        }
        n572 = global read "多参数全局变量.vi" "校准VI引用句柄"() -> (w737:T21)
        n573 = invoke on="探头校准子面板" class="SubPnl" method="Remove VI"() -> (error out=w743:errorcluster)  [unwired: 3 in, 2 out]
        n574 = Bundle By Name(cluster=w737, "ORP校准VI引用句柄"=w735) -> (w736:T21)
        n575 = invoke on="探头校准子面板" class="SubPnl" method="Insert VI"(error in=w743, "VI Ref"=w735) -> ()  [unwired: 2 in, 4 out]
        n576 = global write "多参数全局变量.vi" "校准VI引用句柄"(w736) -> ()
      }
    }
  }
  n577 = property on="编号" class="Str"("Visible"=w27) -> ()  [unwired: 2 in, 2 out]
